vi "MPU_Stick_Read_Write_Configuration.vi"(8 "error in (no error)":errorcluster, 9 "Command":T9, 10 "Configuration Parameter":T10, 11 "MPU_Stick_Globals":T1) -> (0 "error out":errorcluster, 3 "MPU_Stick_Globals Out":T1)   [LabVIEW 2017]
uses:
  Controls/MPU_Stick_Globals.ctl
  Controls/IMU_Configuration_References.ctl
  Controls/MP_Comp_Filter_Constants_References.ctl
  Controls/MD_Threshold_References.ctl
  Controls/MD_Type_References.ctl
  Controls/LED_Configuration_References.ctl
  Controls/Primary_References.ctl
  Controls/MPU_Stick_Queues.ctl
  Controls/MPU_Stick_Queue_Element.ctl
  Controls/MPU_Stick_Queue_Commands.ctl
  Classes/ADCP.lvclass
  Controls/MPU_Stick_Config_Parameters.ctl
  Controls/MPU_Stick_Read_Write_Configurations_Command.ctl
panel:
  out "Parameter Value":string
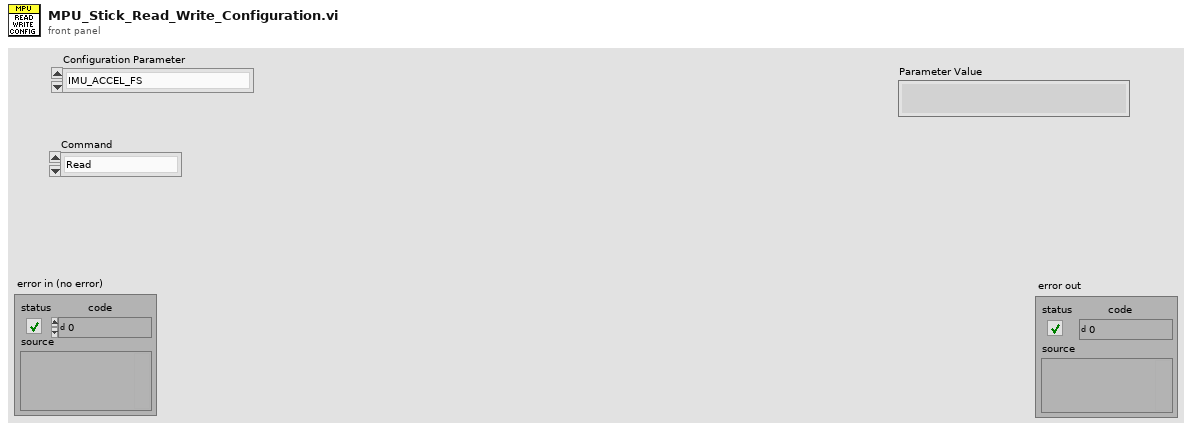
[diagram p1: front panel]
types:
  T1 = typedef "MPU_Stick_Globals.ctl" = cluster{"IMU_configuration_references":T2, "MP_Comp_Filter_Constants_References":T3, "MD_Threshold_References":T4, "MD_Type_References":T5, "LED_Configuration_References":T6, "Primary_references":T7, "MPU_Stick_Queues":T8, "ADCP":refnum<vi>}
  T2 = typedef "IMU_Configuration_References.ctl" = cluster{"Get all IMU configurations":refnum<vi>, "Set all IMU configurations":refnum<vi>, "Get sampling frequency":refnum<vi>, "Set sampling frequency":refnum<vi>, "Get calibration point count":refnum<vi>, "Set calibration point count":refnum<vi>, "Get calibration interval":refnum<vi>, "Set calibration interval":refnum<vi>, "Get Gyroscope bandwidth":refnum<vi>, "Set Gyroscope bandwidth":refnum<vi>, "Get Gyroscope F.S. Value":refnum<vi>, "Set Gyroscope F.S. Value":refnum<vi>, "Get Accelerometer bandwidth":refnum<vi>, "Set Accelerometer bandwidth":refnum<vi>, "Get Accelerometer F.S. Value":refnum<vi>, "Set Accelerometer F.S. Value":refnum<vi>, "Sampling frequency (Hz)":refnum<vi>, "Calibration point count":refnum<vi>, "Calibration interval (ms)":refnum<vi>, "IMU Gyroscope bandwidth":refnum<vi>, "IMU Gyroscope F.S. value":refnum<vi>, "IMU Accelerometer bandwidth":refnum<vi>, "IMU Accelerometer F.S. value":refnum<vi>}
  T3 = typedef "MP_Comp_Filter_Constants_References.ctl" = cluster{"Set pitch filter constant":refnum<vi>, "Get pitch filter constant":refnum<vi>, "Set roll filter constant":refnum<vi>, "Get roll filter constant":refnum<vi>, "Pitch filter constant":refnum<vi>, "Roll filter constant":refnum<vi>}
  T4 = typedef "MD_Threshold_References.ctl" = cluster{"Yaw threshold (U)":refnum<vi>, "Yaw threshold (L)":refnum<vi>, "Pitch threshold (U)":refnum<vi>, "Pitch. threshold (L)":refnum<vi>, "Roll threshold (U)":refnum<vi>, "Roll threshold (L)":refnum<vi>, "Z gyro. threshold (U)":refnum<vi>, "Z gyro. threshold (L)":refnum<vi>, "Y gyro. threshold (U)":refnum<vi>, "Y gyro. threshold (L)":refnum<vi>, "X gyro. threshold (U)":refnum<vi>, "X gyro. threshold (L)":refnum<vi>, "Z accel. threshold (U)":refnum<vi>, "Z accel. threshold (L)":refnum<vi>, "Y accel. threshold (U)":refnum<vi>, "Y accel. threshold (L)":refnum<vi>, "X accel. threshold (U)":refnum<vi>, "X accel. threshold (L)":refnum<vi>, "Set all Motion detection threshold configurations":refnum<vi>, "Get yaw threshold (upper)":refnum<vi>, "Get yaw threshold (lower)":refnum<vi>, "Get pitch threshold (upper)":refnum<vi>, "Get pitch threshold (lower)":refnum<vi>, "Get roll threshold (upper)":refnum<vi>, "Get roll threshold (lower)":refnum<vi>, "Get Z gyro threshold (upper)":refnum<vi>, "Get Z gyro threshold (lower)":refnum<vi>, "Get Y gyro threshold (upper)":refnum<vi>, "Get Y gyro threshold (lower)":refnum<vi>, "Get X gyro threshold (upper)":refnum<vi>, "Get X gyro threshold (lower)":refnum<vi>, "Get Z accel threshold (upper)":refnum<vi>, "Get Z accel threshold (lower)":refnum<vi>, "Get Y accel threshold (upper)":refnum<vi>, "Get Y accel threshold (lower)":refnum<vi>, "Get X accel threshold (upper)":refnum<vi>, "Get X accel threshold (lower)":refnum<vi>, "Get all Motion detection threshold configurations":refnum<vi>, "Set yaw threshold (upper)":refnum<vi>, "Set yaw threshold (lower)":refnum<vi>, "Set pitch threshold (upper)":refnum<vi>, "Set pitch threshold (lower)":refnum<vi>, "Set roll threshold (upper)":refnum<vi>, "Set roll threshold (lower)":refnum<vi>, "Set Z gyro threshold (upper)":refnum<vi>, "Set Z gyro threshold (lower)":refnum<vi>, "Set Y gyro threshold (upper)":refnum<vi>, "Set Y gyro threshold (lower)":refnum<vi>, "Set X gyro threshold (upper)":refnum<vi>, "Set X gyro threshold (lower)":refnum<vi>, "Set Z accel threshold (upper)":refnum<vi>, "Set Z accel threshold (lower)":refnum<vi>, "Set Y accel threshold (upper)":refnum<vi>, "Set Y accel threshold (lower)":refnum<vi>, "Set X accel threshold (upper)":refnum<vi>, "Set X accel threshold (lower)":refnum<vi>}
  T5 = typedef "MD_Type_References.ctl" = cluster{"Yaw threshold type":refnum<vi>, "Pitch threshold type":refnum<vi>, "Roll threshold type":refnum<vi>, "Z gyro threshold type":refnum<vi>, "Y gyro threshold type":refnum<vi>, "X gyro threshold type":refnum<vi>, "Z accel threshold type":refnum<vi>, "Y accel threshold type":refnum<vi>, "X accel threshold type":refnum<vi>, "Set all Motion detection type configurations":refnum<vi>, "Get all Motion detection type configurations":refnum<vi>, "Set yaw threshold type":refnum<vi>, "Get yaw threshold type":refnum<vi>, "Set pitch threshold type":refnum<vi>, "Get pitch threshold type":refnum<vi>, "Set roll threshold type":refnum<vi>, "Get roll threshold type":refnum<vi>, "Set Z gyroscope threshold type":refnum<vi>, "Get Z gyroscope threshold type":refnum<vi>, "Set Y gyroscope threshold type":refnum<vi>, "Get Y gyroscope threshold type":refnum<vi>, "Set X gyroscope threshold type":refnum<vi>, "Get X gyroscope threshold type":refnum<vi>, "Set Z accel threshold type":refnum<vi>, "Get Z accel threshold type":refnum<vi>, "Set Y accel threshold type":refnum<vi>, "Get Y accel threshold type":refnum<vi>, "Get X accel threshold type":refnum<vi>, "Set X accel threshold type":refnum<vi>}
  T6 = typedef "LED_Configuration_References.ctl" = cluster{"Get all LED configurations":refnum<vi>, "Set all LED configurations":refnum<vi>, "Get LED3 configuration":refnum<vi>, "Set LED3 configuration":refnum<vi>, "Get LED2 configuration":refnum<vi>, "Set LED2 configuration":refnum<vi>, "Get LED1 configuration":refnum<vi>, "Set LED1 configuration":refnum<vi>, "LED3 Configuration":refnum<vi>, "LED2 Configuration":refnum<vi>, "LED1 Configuration":refnum<vi>}
  T7 = typedef "Primary_References.ctl" = cluster{"3D View Image":refnum<vi>, "Plot":refnum<vi>, "Graph / 3D view tab control":refnum<vi>, "MP Reset":refnum<vi>, "Calibrate IMU":refnum<vi>, "Plot Parameter List":refnum<vi>, "Remove Parameter from Plot":refnum<vi>, "Add Parameter to Plot":refnum<vi>, "Parameter to monitor":refnum<vi>, "Yaw motion detection output":refnum<vi>, "Pitch motion detection output":refnum<vi>, "Roll motion detection output":refnum<vi>, "Z gyro motion detection output":refnum<vi>, "Y gyro motion detection output":refnum<vi>, "X gyro motion detection output":refnum<vi>, "Z accel motion detection output":refnum<vi>, "Y accel motion detection output":refnum<vi>, "X accel motion detection output":refnum<vi>, "Yaw angle (filter) (degrees)":refnum<vi>, "Pitch angle (filter) (degrees)":refnum<vi>, "Roll angle (filter) (degrees)":refnum<vi>, "Yaw angle (gyro) (degrees)":refnum<vi>, "Pitch angle (gyro) (degrees)":refnum<vi>, "Roll angle (gyro) (degrees)":refnum<vi>, "Yaw angle (accel) (degrees)":refnum<vi>, "Pitch angle (accel) (degrees)":refnum<vi>, "Roll angle (accel) (degrees)":refnum<vi>, "Z gyroscope reading (DPS)":refnum<vi>, "Y gyroscope reading (DPS)":refnum<vi>, "X gyroscope reading (DPS)":refnum<vi>, "Z accelerometer reading (G)":refnum<vi>, "Y accelerometer reading (G)":refnum<vi>, "X accelerometer reading (G)":refnum<vi>, "Save all config.":refnum<vi>, "Write all config.":refnum<vi>, "Read all config.":refnum<vi>, "Tab Control":refnum<vi>, "Baud Rate":refnum<vi>, "COM Port":refnum<vi>, "Time (ms)":refnum<vi>, "Value (Units)":refnum<vi>, "Exit Application":refnum<vi>, "Connect Device":refnum<vi>, "Progress Bar":refnum<vi>, "Get Range & Offset":refnum<vi>, "Range":refnum<vi>, "Offset":refnum<vi>, "Set Range & Offset":refnum<vi>, "Parameter name":refnum<vi>, "Plot time (ms)":refnum<vi>, "Plot value":refnum<vi>}
  T8 = typedef "MPU_Stick_Queues.ctl" = cluster{"UI Event Handler":refnum<queue>, "3D View Updater":refnum<queue>, "Plot Updater":refnum<queue>, "Serial Port Reader":refnum<queue>, "UI Indicators Updater":refnum<queue>}
  T9 = typedef "MPU_Stick_Read_Write_Configurations_Command.ctl" = enum16{"Read", "Write", "Write All", "Read All"}
  T10 = typedef "MPU_Stick_Config_Parameters.ctl" = enum16{"IMU_ACCEL_FS", "IMU_ACCEL_BW", "IMU_GYRO_FS", "IMU_GYRO_BW", "IMU_CALIB_INTERVAL", "IMU_CALIB_POINT_COUNT", "IMU_SAMPLING_FREQ", "LED1_CONFIG", "LED2_CONFIG", "LED3_CONFIG", "MP_ROLL_FILTER_CONSTANT", "MP_PITCH_FILTER_CONSTANT", "MP_THRESHOLD_X_ACCEL_LOW", "MP_THRESHOLD_X_ACCEL_HIGH", "MP_THRESHOLD_Y_ACCEL_LOW", "MP_THRESHOLD_Y_ACCEL_HIGH", "MP_THRESHOLD_Z_ACCEL_LOW", "MP_THRESHOLD_Z_ACCEL_HIGH", "MP_THRESHOLD_X_GYRO_LOW", "MP_THRESHOLD_X_GYRO_HIGH", "MP_THRESHOLD_Y_GYRO_LOW", "MP_THRESHOLD_Y_GYRO_HIGH", "MP_THRESHOLD_Z_GYRO_LOW", "MP_THRESHOLD_Z_GYRO_HIGH", "MP_THRESHOLD_ROLL_LOW", "MP_THRESHOLD_ROLL_HIGH", "MP_THRESHOLD_PITCH_LOW", "MP_THRESHOLD_PITCH_HIGH", "MP_THRESHOLD_YAW_LOW", "MP_THRESHOLD_YAW_HIGH", "MP_DETECTION_TYPE_X_ACCEL", "MP_DETECTION_TYPE_Y_ACCEL", "MP_DETECTION_TYPE_Z_ACCEL", "MP_DETECTION_TYPE_X_GYRO", "MP_DETECTION_TYPE_Y_GYRO", "MP_DETECTION_TYPE_Z_GYRO", "MP_DETECTION_TYPE_ROLL", "MP_DETECTION_TYPE_PITCH", "MP_DETECTION_TYPE_YAW"}
  T11 = cluster{"Parameter name":string, "Node name":string, "Node ID":u8, "Frame name":string, "Frame ID":u8, "Start bit":u32, "Bit length":u32, "Factor":dbl, "Offset":dbl, "Minimum":dbl, "Maximum":dbl, "Value":string, "Comments":string, "Data_Type":enum16{"BOOL", "UNSIGNED", "SIGNED", "FLOAT32", "ENUM"}, "Enum List":string[]}[]
  T12 = typedef "IMU_Accelerometer_Full_Scale_Values.ctl" = enum16{"2G", "4G", "8G", "16G"}
  T13 = typedef "IMU_Accelerometer_Bandwidth.ctl" = enum16{"IMU_ACCEL_BW_460_Hz", "IMU_ACCEL_BW_184_Hz", "IMU_ACCEL_BW_92_Hz", "IMU_ACCEL_BW_41_Hz", "IMU_ACCEL_BW_20_Hz", "IMU_ACCEL_BW_10_Hz", "IMU_ACCEL_BW_5_Hz"}
  T14 = typedef "IMU_Gyroscope_Full_Scale_Values.ctl" = enum16{"250 DPS", "500 DPS", "1000 DPS", "2000 DPS"}
  T15 = typedef "IMU_Gyroscope_Bandwidth.ctl" = enum16{"IMU_GYRO_BW_NONE", "IMU_GYRO_BW_184_Hz", "IMU_GYRO_BW_92_Hz", "IMU_GYRO_BW_41_Hz", "IMU_GYRO_BW_20_Hz", "IMU_GYRO_BW_10_Hz", "IMU_GYRO_BW_5_Hz"}
  T16 = typedef "LED_config.ctl" = enum16{"UC_DIGITAL_OUTPUT", "X_ACCEL_PWM", "Y_ACCEL_PWM", "Z_ACCEL_PWM", "X_ACCEL_MD_OUTPUT", "Y_ACCEL_MD_OUTPUT", "Z_ACCEL_MD_OUTPUT", "X_GYRO_PWM", "Y_GYRO_PWM", "Z_GYRO_PWM", "X_GYRO_MD_OUTPUT", "Y_GYRO_MD_OUTPUT", "Z_GYRO_MD_OUTPUT", "ROLL_PWM_OUTPUT", "PITCH_PWM_OUTPUT", "YAW_PWM_OUTPUT", "ROLL_MD_OUTPUT", "PITCH_MD_OUTPUT", "YAW_MD_OUTPUT", "UC_PWM_OUTPUT"}
  T17 = typedef "Motion_Detection_Threshold_Type.ctl" = enum16{"ABS_LESSER_THAN", "ABS_GREATER_THAN", "LESSER_THAN", "GREATER_THAN", "WINDOWED_MODE_WITHIN_BOUNDS", "WINDOWED_MODE_OUTSIDE_BOUNDS"}
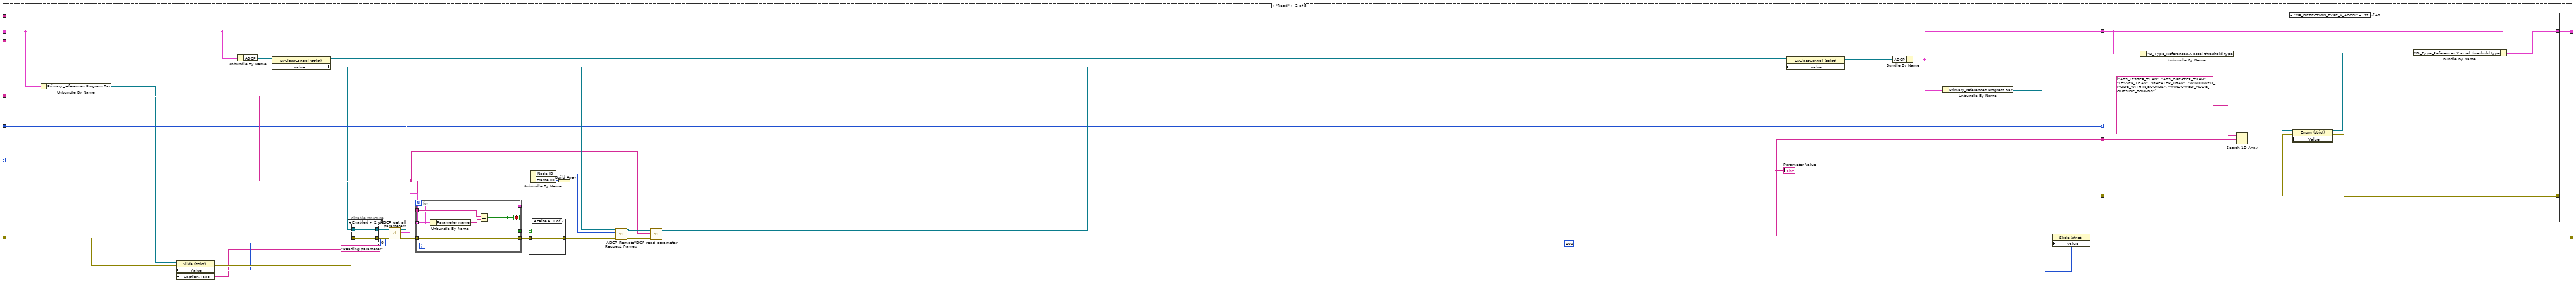
[diagram p4: hidden frame]
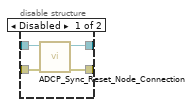
[diagram p5: hidden frame]
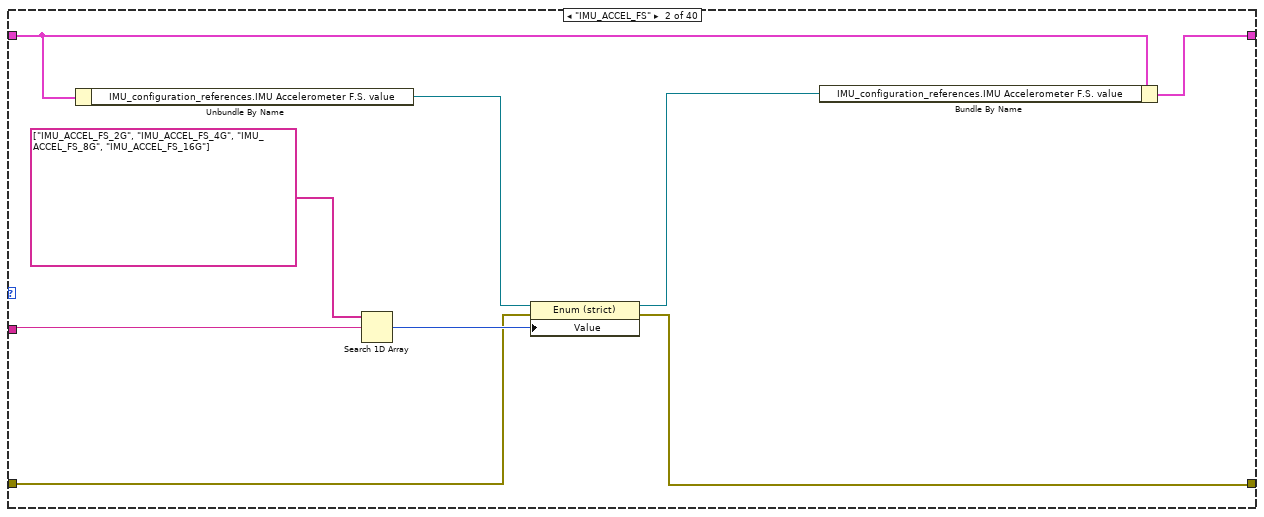
[diagram p8: hidden frame]
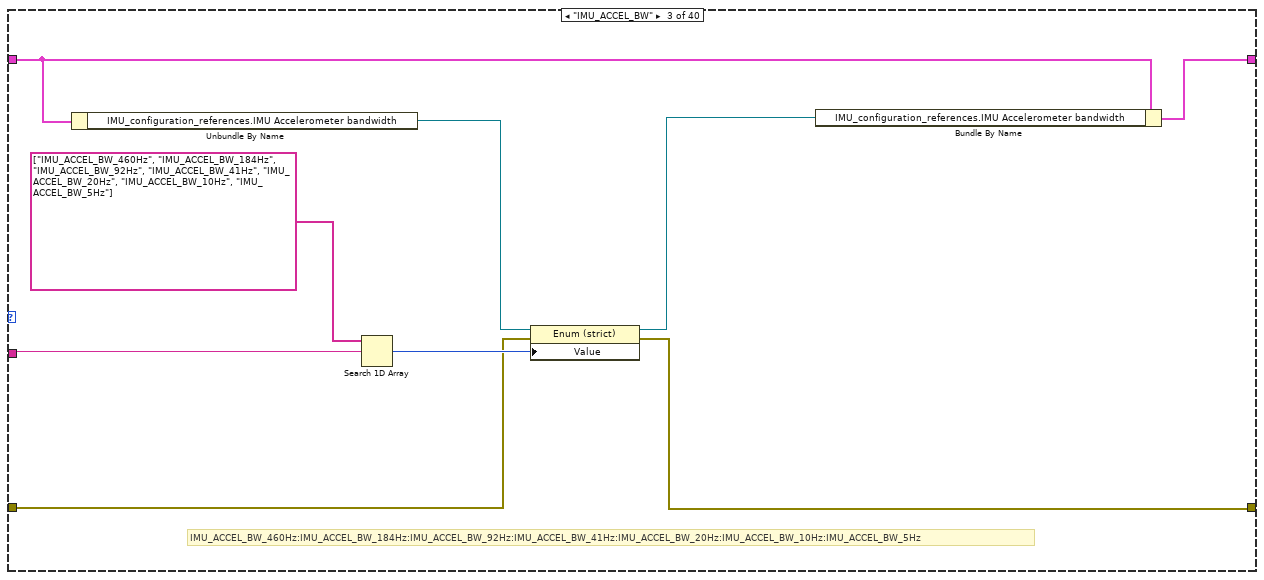
[diagram p9: hidden frame]
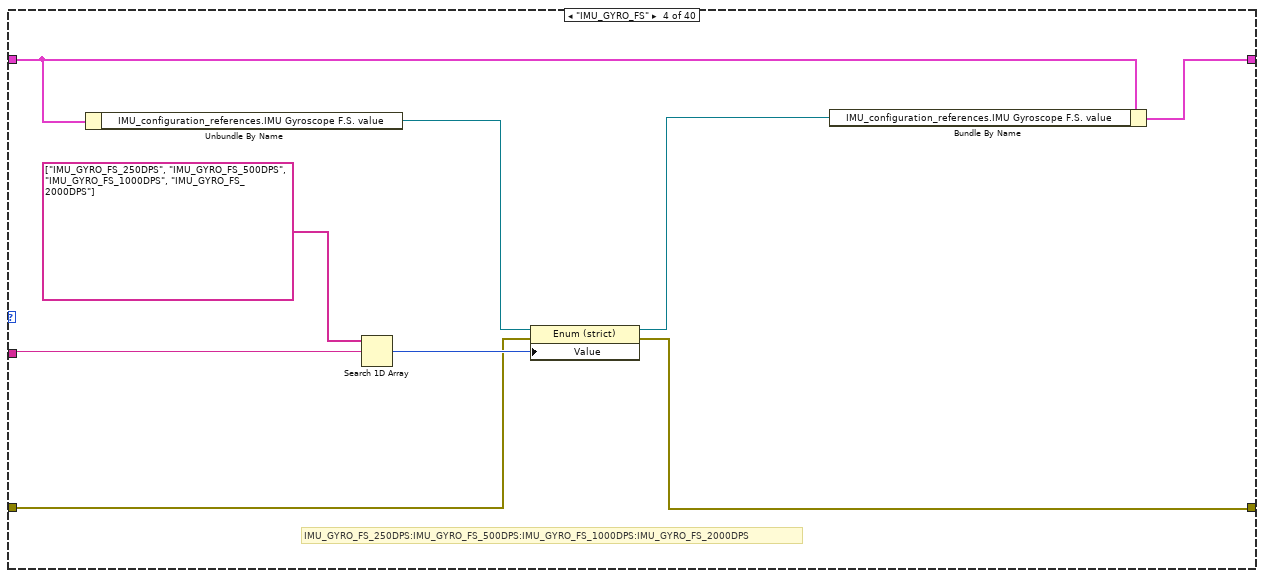
[diagram p10: hidden frame]
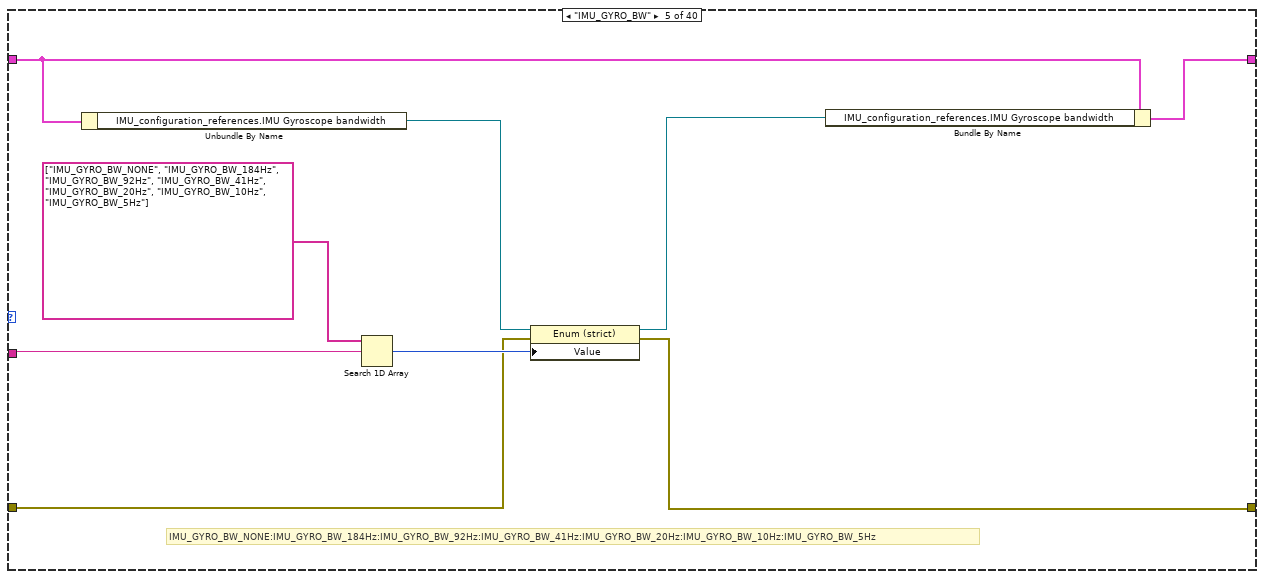
[diagram p11: hidden frame]
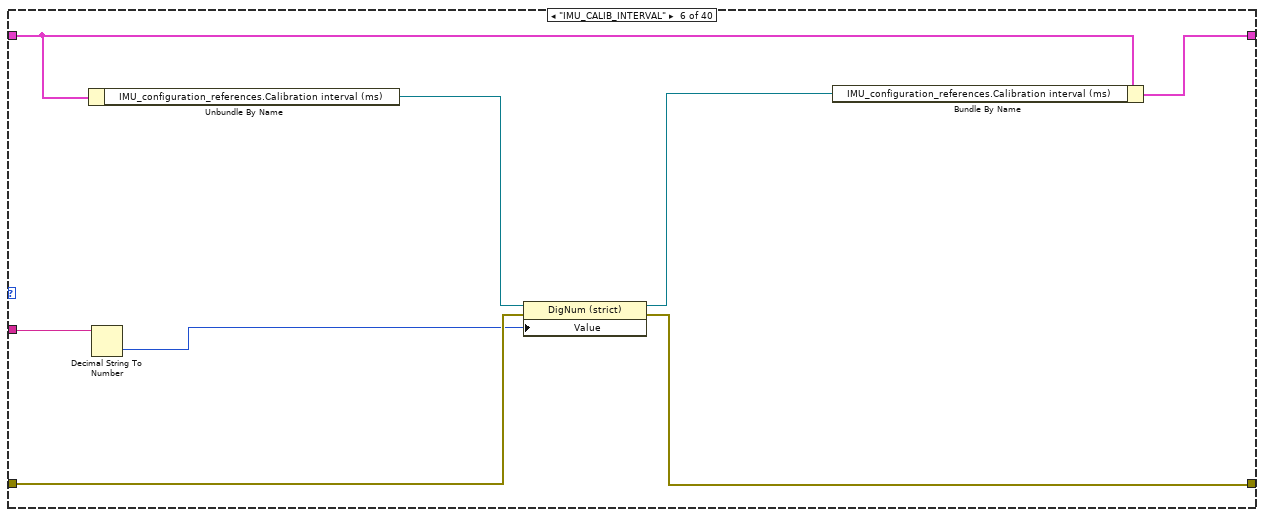
[diagram p12: hidden frame]
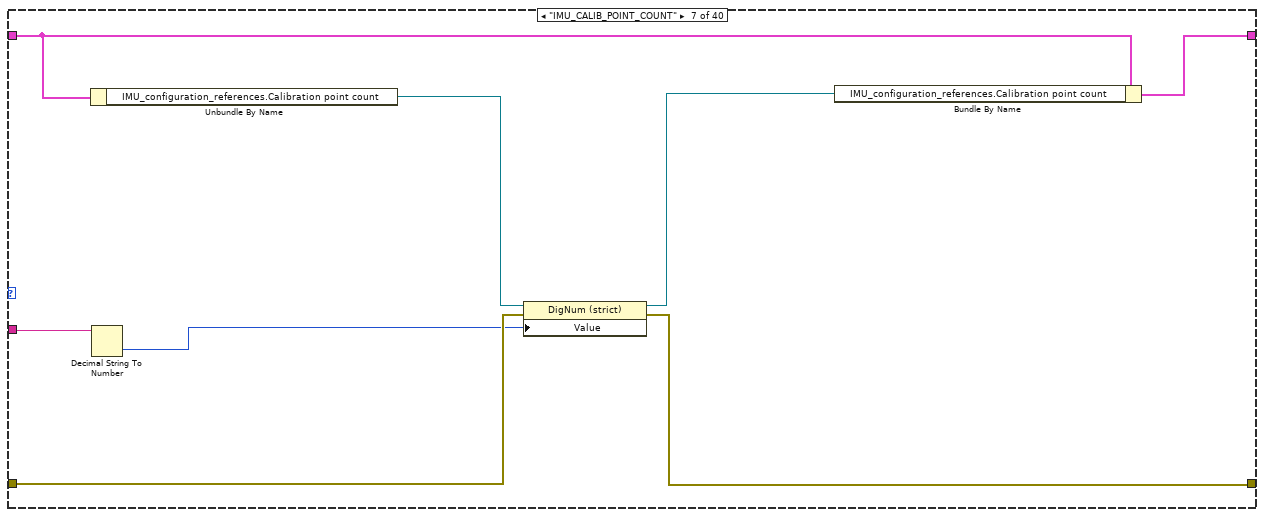
[diagram p13: hidden frame]
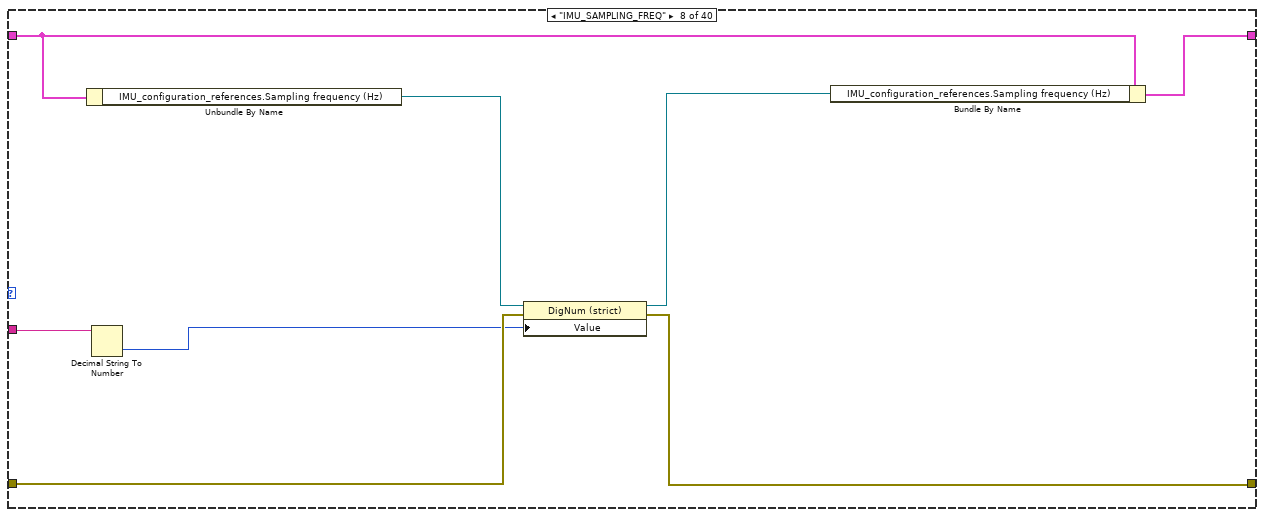
[diagram p14: hidden frame]
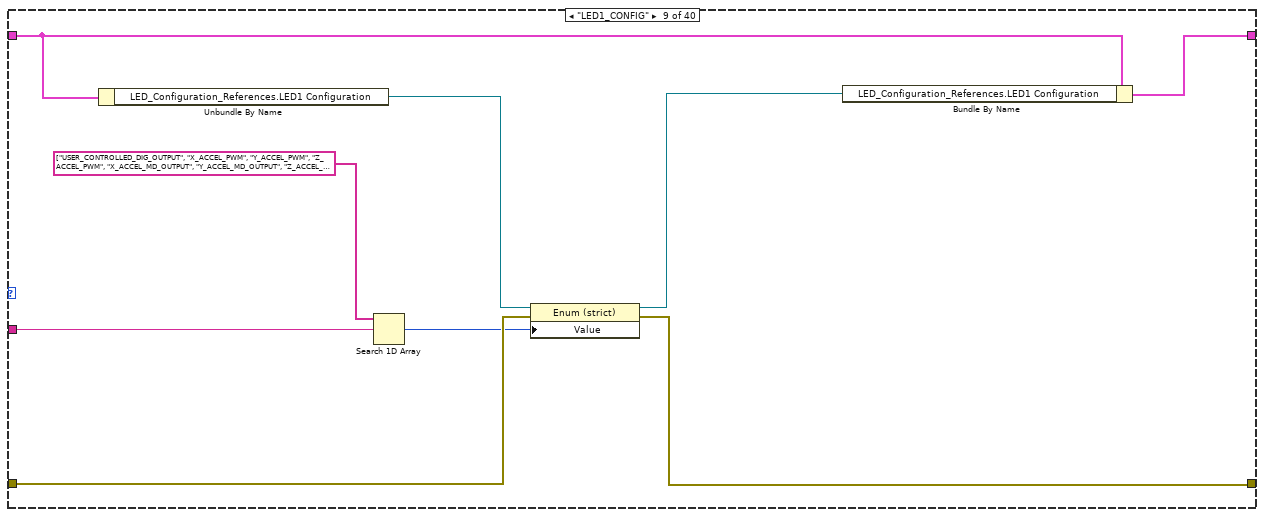
[diagram p15: hidden frame]
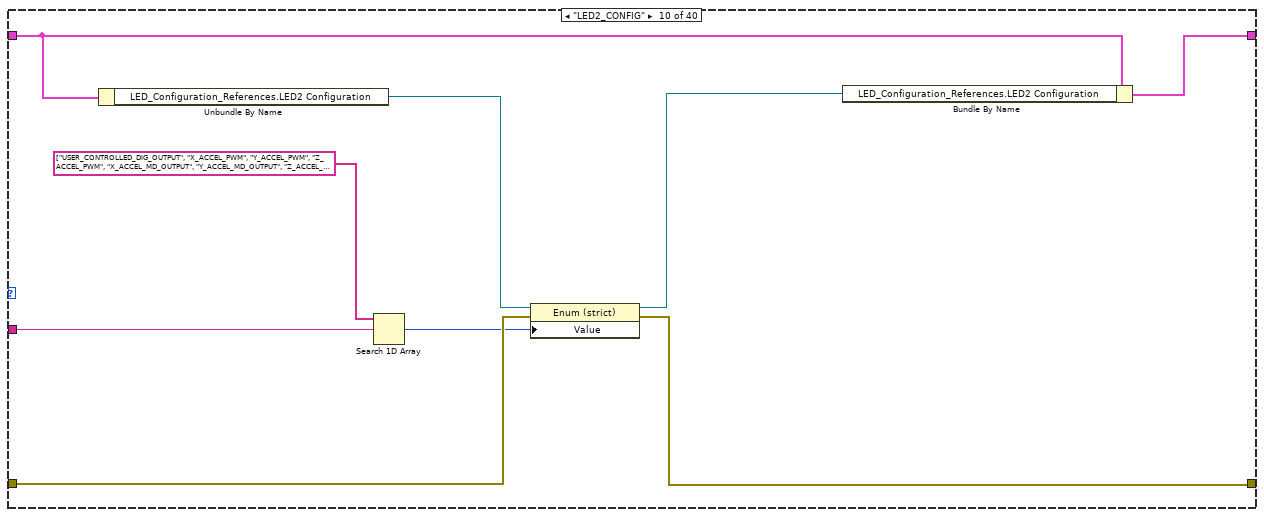
[diagram p16: hidden frame]
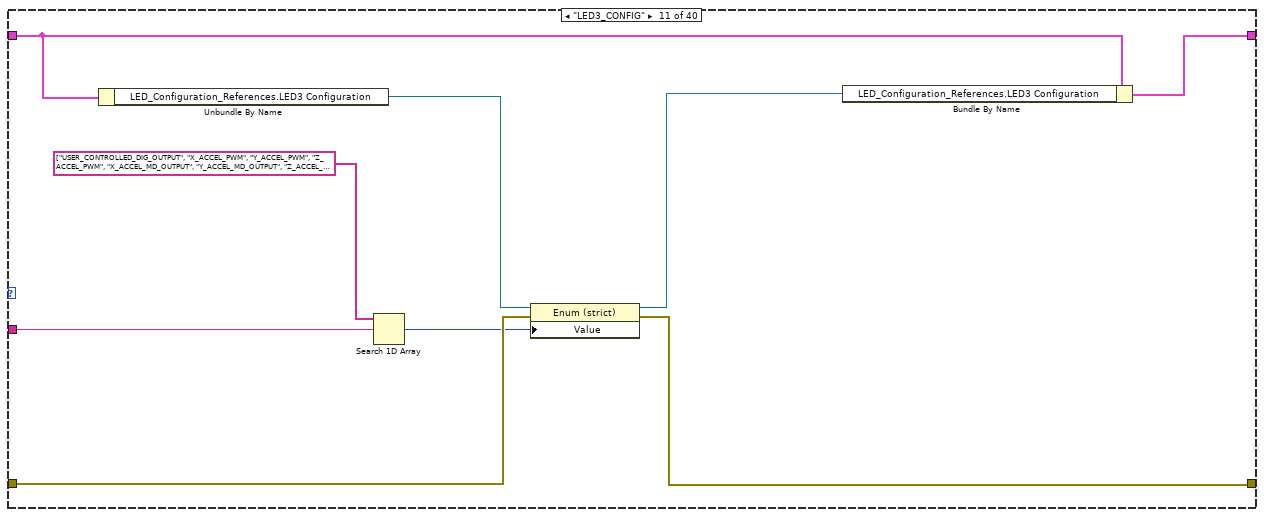
[diagram p17: hidden frame]
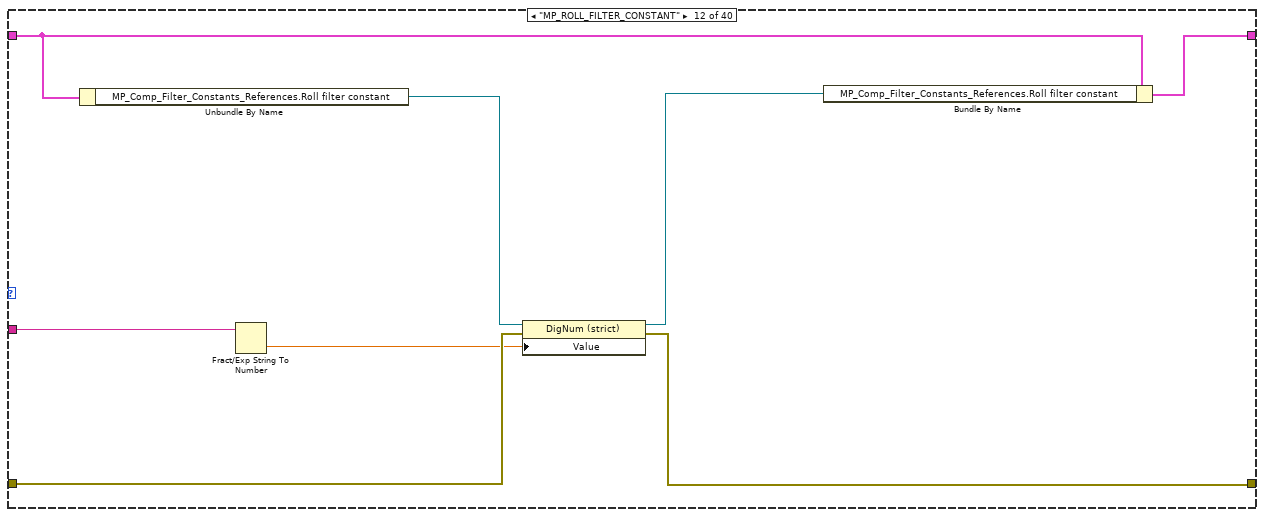
[diagram p18: hidden frame]
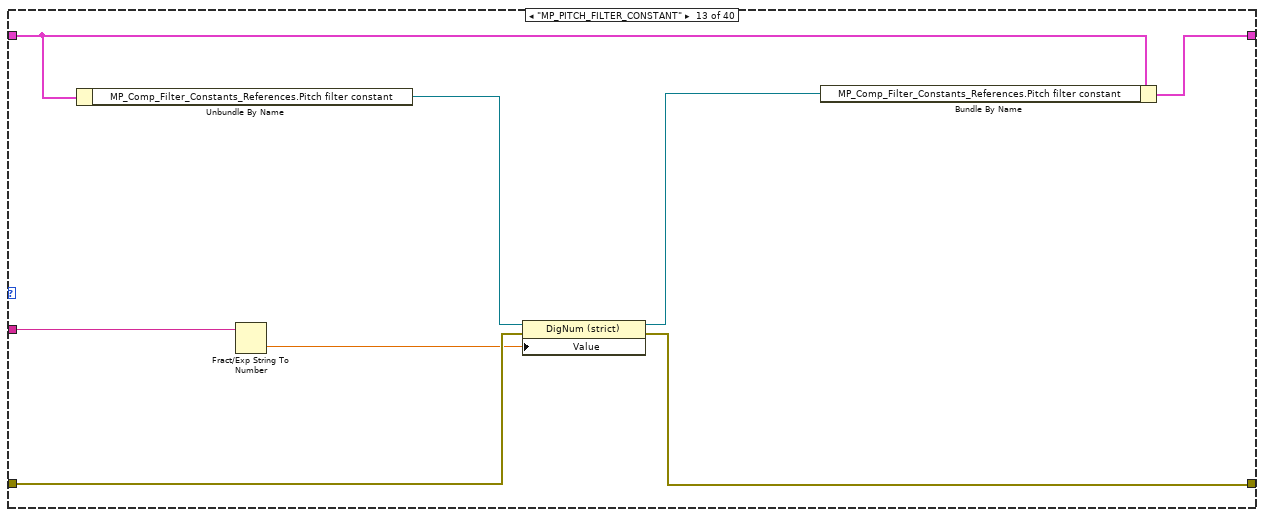
[diagram p19: hidden frame]
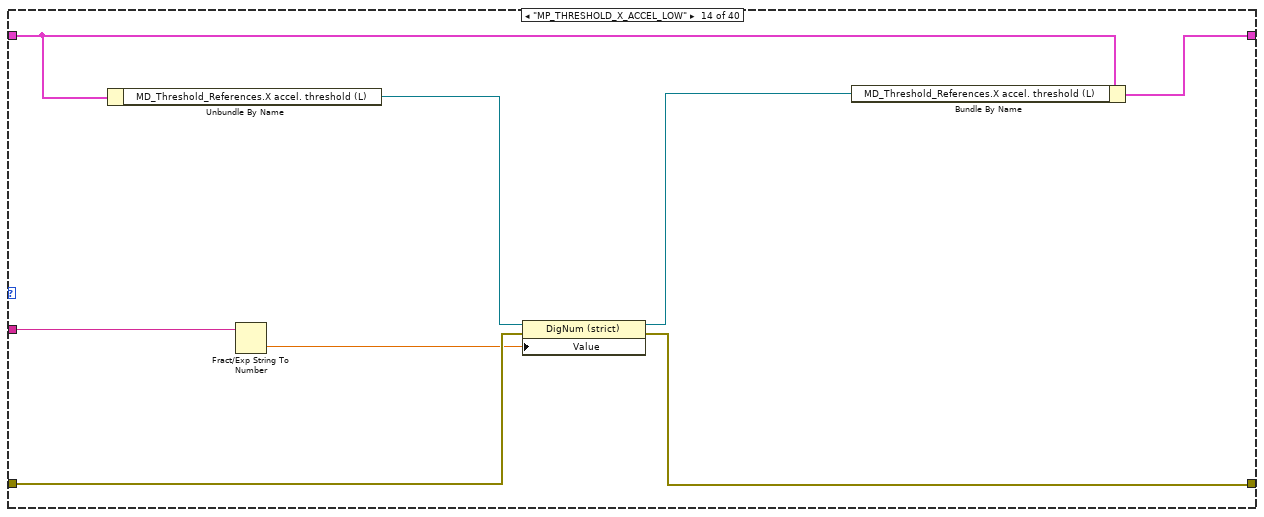
[diagram p20: hidden frame]
diagram:
  (unwired) string[] ["MPU_STICK:IMU_CONFIG_WRITE_ENABLE:IMU_CONFIG_ACCEL_FS_WE", "MPU_STICK:IMU_CONFIG_WRITE_ENABLE:IMU_CONFIG_ACCEL_BW_WE", "MPU_STICK:IMU_CONFIG_WRITE_ENABLE:IMU_CONFIG_GYRO_FS_WE", "MPU_STICK:IMU_CONFIG_WRITE_ENABLE:IMU_CONFIG_GYRO_BW_WE", "MPU_STICK:IMU_CONFIG_WRITE_ENABLE:IMU_CONFIG_CALIB_INTERVAL_WE", "MPU_STICK:IMU_CONFIG_WRITE_ENABLE:IMU_CONFIG_CALIB_POINTS_WE", "MPU_STICK:IMU_CONFIG_WRITE_ENABLE:IMU_CONFIG_SAMPLING_RATE_WE", "MPU_STICK:LED_MODE_CONFIG:LED1_MODE_WE", "MPU_STICK:LED_MODE_CONFIG:LED2_MODE_WE", "MPU_STICK:LED_MODE_CONFIG:LED3_MODE_WE", "MPU_STICK:MD_WRITE_CONFIG:MP_ROLL_FILTER_CONSTANT_WE", "MPU_STICK:MD_WRITE_CONFIG:MP_PITCH_FILTER_CONSTANT_WE", "MPU_STICK:MD_WRITE_CONFIG:MD_ACCEL_X_THRESHOLD_LOW_WE", "MPU_STICK:MD_WRITE_CONFIG:MD_ACCEL_X_THRESHOLD_HIGH_WE", "MPU_STICK:MD_WRITE_CONFIG:MD_ACCEL_Y_THRESHOLD_LOW_WE", "MPU_STICK:MD_WRITE_CONFIG:MD_ACCEL_Y_THRESHOLD_HIGH_WE", "MPU_STICK:MD_WRITE_CONFIG:MD_ACCEL_Z_THRESHOLD_LOW_WE", "MPU_STICK:MD_WRITE_CONFIG:MD_ACCEL_Z_THRESHOLD_HIGH_WE", "MPU_STICK:MD_WRITE_CONFIG:MD_GYRO_X_THRESHOLD_LOW_WE", "MPU_STICK:MD_WRITE_CONFIG:MD_GYRO_X_THRESHOLD_HIGH_WE", "MPU_STICK:MD_WRITE_CONFIG:MD_GYRO_Y_THRESHOLD_LOW_WE", "MPU_STICK:MD_WRITE_CONFIG:MD_GYRO_Y_THRESHOLD_HIGH_WE", "MPU_STICK:MD_WRITE_CONFIG:MD_GYRO_Z_THRESHOLD_LOW_WE", "MPU_STICK:MD_WRITE_CONFIG:MD_GYRO_Z_THRESHOLD_HIGH_WE", "MPU_STICK:MD_WRITE_CONFIG:MD_ROLL_THRESHOLD_LOW_WE", "MPU_STICK:MD_WRITE_CONFIG:MD_ROLL_THRESHOLD_HIGH_WE", "MPU_STICK:MD_WRITE_CONFIG:MD_PITCH_THRESHOLD_LOW_WE", "MPU_STICK:MD_WRITE_CONFIG:MD_PITCH_THRESHOLD_HIGH_WE", "MPU_STICK:MD_WRITE_CONFIG:MD_YAW_THRESHOLD_LOW_WE", "MPU_STICK:MD_WRITE_CONFIG:MD_YAW_THRESHOLD_HIGH_WE", "MPU_STICK:MD_WRITE_CONFIG:MD_ACCEL_X_THRESHOLD_TYPE_WE", "MPU_STICK:MD_WRITE_CONFIG:MD_ACCEL_Y_THRESHOLD_TYPE_WE", "MPU_STICK:MD_WRITE_CONFIG:MD_ACCEL_Z_THRESHOLD_TYPE_WE", "MPU_STICK:MD_WRITE_CONFIG:MD_GYRO_X_THRESHOLD_TYPE_WE", "MPU_STICK:MD_WRITE_CONFIG:MD_GYRO_Y_THRESHOLD_TYPE_WE", "MPU_STICK:MD_WRITE_CONFIG:MD_GYRO_Z_THRESHOLD_TYPE_WE", "MPU_STICK:MD_WRITE_CONFIG:MD_ROLL_THRESHOLD_TYPE_WE", "MPU_STICK:MD_WRITE_CONFIG:MD_PITCH_THRESHOLD_TYPE_WE", "MPU_STICK:MD_WRITE_CONFIG:MD_YAW_THRESHOLD_TYPE_WE"]  # MPU Stick Configuration Write Enable Bit Names
  (unwired) string[] ["MPU_STICK:IMU_CONFIG_REG_B:IMU_CONFIG_ACCEL_FS", "MPU_STICK:IMU_CONFIG_REG_B:IMU_CONFIG_ACCEL_BW", "MPU_STICK:IMU_CONFIG_REG_B:IMU_CONFIG_GYRO_FS", "MPU_STICK:IMU_CONFIG_REG_B:IMU_CONFIG_GYRO_BW", "MPU_STICK:IMU_CONFIG_REG_A:IMU_CONFIG_CALIB_INTERVAL", "MPU_STICK:IMU_CONFIG_REG_A:IMU_CONFIG_CALIB_POINTS", "MPU_STICK:IMU_CONFIG_REG_A:IMU_CONFIG_SAMPLING_RATE", "MPU_STICK:LED_MODE_CONFIG:LED1_MODE", "MPU_STICK:LED_MODE_CONFIG:LED2_MODE", "MPU_STICK:LED_MODE_CONFIG:LED3_MODE", "MPU_STICK:MP_ROLL_FILTER_CONSTANT:MP_ROLL_FILTER_CONSTANT", "MPU_STICK:MP_PITCH_FILTER_CONSTANT:MP_PITCH_FILTER_CONSTANT", "MPU_STICK:MD_ACCEL_X_THRESHOLD_LOW:MD_ACCEL_X_THRESHOLD_LOW", "MPU_STICK:MD_ACCEL_X_THRESHOLD_HIGH:MD_ACCEL_X_THRESHOLD_HIGH", "MPU_STICK:MD_ACCEL_Y_THRESHOLD_LOW:MD_ACCEL_Y_THRESHOLD_LOW", "MPU_STICK:MD_ACCEL_Y_THRESHOLD_HIGH:MD_ACCEL_Y_THRESHOLD_HIGH", "MPU_STICK:MD_ACCEL_Z_THRESHOLD_LOW:MD_ACCEL_Z_THRESHOLD_LOW", "MPU_STICK:MD_ACCEL_Z_THRESHOLD_HIGH:MD_ACCEL_Z_THRESHOLD_HIGH", "MPU_STICK:MD_GYRO_X_THRESHOLD_LOW:MD_GYRO_X_THRESHOLD_LOW", "MPU_STICK:MD_GYRO_X_THRESHOLD_HIGH:MD_GYRO_X_THRESHOLD_HIGH", "MPU_STICK:MD_GYRO_Y_THRESHOLD_LOW:MD_GYRO_Y_THRESHOLD_LOW", "MPU_STICK:MD_GYRO_Y_THRESHOLD_HIGH:MD_GYRO_Y_THRESHOLD_HIGH", "MPU_STICK:MD_GYRO_Z_THRESHOLD_LOW:MD_GYRO_Z_THRESHOLD_LOW", "MPU_STICK:MD_GYRO_Z_THRESHOLD_HIGH:MD_GYRO_Z_THRESHOLD_HIGH", "MPU_STICK:MD_ROLL_THRESHOLD_LOW:MD_ROLL_THRESHOLD_LOW", "MPU_STICK:MD_ROLL_THRESHOLD_HIGH:MD_ROLL_THRESHOLD_HIGH", "MPU_STICK:MD_PITCH_THRESHOLD_LOW:MD_PITCH_THRESHOLD_LOW", "MPU_STICK:MD_PITCH_THRESHOLD_HIGH:MD_PITCH_THRESHOLD_HIGH", "MPU_STICK:MD_YAW_THRESHOLD_LOW:MD_YAW_THRESHOLD_LOW", "MPU_STICK:MD_YAW_THRESHOLD_HIGH:MD_YAW_THRESHOLD_HIGH", "MPU_STICK:MD_THRESHOLD_TYPE:MD_ACCEL_X_THRESHOLD_TYPE", "MPU_STICK:MD_THRESHOLD_TYPE:MD_ACCEL_Y_THRESHOLD_TYPE", "MPU_STICK:MD_THRESHOLD_TYPE:MD_ACCEL_Z_THRESHOLD_TYPE", "MPU_STICK:MD_THRESHOLD_TYPE:MD_GYRO_X_THRESHOLD_TYPE", "MPU_STICK:MD_THRESHOLD_TYPE:MD_GYRO_Y_THRESHOLD_TYPE", "MPU_STICK:MD_THRESHOLD_TYPE:MD_GYRO_Z_THRESHOLD_TYPE", "MPU_STICK:MD_THRESHOLD_TYPE:MD_ROLL_THRESHOLD_TYPE", "MPU_STICK:MD_THRESHOLD_TYPE:MD_PITCH_THRESHOLD_TYPE", "MPU_STICK:MD_THRESHOLD_TYPE:MD_YAW_THRESHOLD_TYPE"]  # MPU Stick Configuration Parameters
  (unwired) string[] ["MPU_STICK:IMU_CONFIG_WRITE_ENABLE:IMU_CONFIG_SAMPLING_RATE_WE", "MPU_STICK:IMU_CONFIG_WRITE_ENABLE:IMU_CONFIG_CALIB_INTERVAL_WE", "MPU_STICK:IMU_CONFIG_WRITE_ENABLE:IMU_CONFIG_CALIB_POINTS_WE", "MPU_STICK:IMU_CONFIG_WRITE_ENABLE:IMU_CONFIG_GYRO_BW_WE", "MPU_STICK:IMU_CONFIG_WRITE_ENABLE:IMU_CONFIG_ACCEL_BW_WE", "MPU_STICK:IMU_CONFIG_WRITE_ENABLE:IMU_CONFIG_GYRO_FS_WE", "MPU_STICK:IMU_CONFIG_WRITE_ENABLE:IMU_CONFIG_ACCEL_FS_WE", "MPU_STICK:MD_WRITE_CONFIG:MD_ACCEL_X_THRESHOLD_LOW_WE", "MPU_STICK:MD_WRITE_CONFIG:MD_ACCEL_X_THRESHOLD_HIGH_WE", "MPU_STICK:MD_WRITE_CONFIG:MD_ACCEL_Y_THRESHOLD_LOW_WE", "MPU_STICK:MD_WRITE_CONFIG:MD_ACCEL_Y_THRESHOLD_HIGH_WE", "MPU_STICK:MD_WRITE_CONFIG:MD_ACCEL_Z_THRESHOLD_LOW_WE", "MPU_STICK:MD_WRITE_CONFIG:MD_ACCEL_Z_THRESHOLD_HIGH_WE", "MPU_STICK:MD_WRITE_CONFIG:MD_GYRO_X_THRESHOLD_LOW_WE", "MPU_STICK:MD_WRITE_CONFIG:MD_GYRO_X_THRESHOLD_HIGH_WE", "MPU_STICK:MD_WRITE_CONFIG:MD_GYRO_Y_THRESHOLD_LOW_WE", "MPU_STICK:MD_WRITE_CONFIG:MD_GYRO_Y_THRESHOLD_HIGH_WE", "MPU_STICK:MD_WRITE_CONFIG:MD_GYRO_Z_THRESHOLD_LOW_WE", "MPU_STICK:MD_WRITE_CONFIG:MD_GYRO_Z_THRESHOLD_HIGH_WE", "MPU_STICK:MD_WRITE_CONFIG:MD_ROLL_THRESHOLD_LOW_WE", "MPU_STICK:MD_WRITE_CONFIG:MD_ROLL_THRESHOLD_HIGH_WE", "MPU_STICK:MD_WRITE_CONFIG:MD_PITCH_THRESHOLD_LOW_WE", "MPU_STICK:MD_WRITE_CONFIG:MD_PITCH_THRESHOLD_HIGH_WE", "MPU_STICK:MD_WRITE_CONFIG:MD_YAW_THRESHOLD_LOW_WE", "MPU_STICK:MD_WRITE_CONFIG:MD_YAW_THRESHOLD_HIGH_WE", "MPU_STICK:MD_WRITE_CONFIG:MP_ROLL_FILTER_CONSTANT_WE", "MPU_STICK:MD_WRITE_CONFIG:MP_PITCH_FILTER_CONSTANT_WE", "MPU_STICK:MD_WRITE_CONFIG:MP_YAW_FILTER_CONSTANT_WE", "MPU_STICK:MD_WRITE_CONFIG:MD_ACCEL_X_THRESHOLD_TYPE_WE", "MPU_STICK:MD_WRITE_CONFIG:MD_ACCEL_Y_THRESHOLD_TYPE_WE", "MPU_STICK:MD_WRITE_CONFIG:MD_ACCEL_Z_THRESHOLD_TYPE_WE", "MPU_STICK:MD_WRITE_CONFIG:MD_GYRO_X_THRESHOLD_TYPE_WE", "MPU_STICK:MD_WRITE_CONFIG:MD_GYRO_Y_THRESHOLD_TYPE_WE", "MPU_STICK:MD_WRITE_CONFIG:MD_GYRO_Z_THRESHOLD_TYPE_WE", "MPU_STICK:MD_WRITE_CONFIG:MD_ROLL_THRESHOLD_TYPE_WE", "MPU_STICK:MD_WRITE_CONFIG:MD_PITCH_THRESHOLD_TYPE_WE", "MPU_STICK:MD_WRITE_CONFIG:MD_YAW_THRESHOLD_TYPE_WE", "MPU_STICK:LED_MODE_CONFIG:LED1_MODE_WE", "MPU_STICK:LED_MODE_CONFIG:LED2_MODE_WE", "MPU_STICK:LED_MODE_CONFIG:LED3_MODE_WE", "MPU_STICK:LED_UC_WRITE:LED_UC_STATE_WE", "MPU_STICK:LED_UC_WRITE:LED_UC_DUTY_WE"] ("Array")
  n1 = while {
    shift-right: [w14] -> w1
    shift-left: "MPU_Stick_Globals" -> [w15]
    tunnel: "Configuration Parameter" -> [w8]
    tunnel: "error in (no error)" -> [w13]
    tunnel: "Command" -> [w16]
    tunnel: [w12] -> w2
    stop <- TRUE stop-if-true
    w9 = string[] ["MPU_STICK:IMU_CONFIG_WRITE_ENABLE:IMU_CONFIG_ACCEL_FS_WE", "MPU_STICK:IMU_CONFIG_WRITE_ENABLE:IMU_CONFIG_ACCEL_BW_WE", "MPU_STICK:IMU_CONFIG_WRITE_ENABLE:IMU_CONFIG_GYRO_FS_WE", "MPU_STICK:IMU_CONFIG_WRITE_ENABLE:IMU_CONFIG_GYRO_BW_WE", "MPU_STICK:IMU_CONFIG_WRITE_ENABLE:IMU_CONFIG_CALIB_INTERVAL_WE", "MPU_STICK:IMU_CONFIG_WRITE_ENABLE:IMU_CONFIG_CALIB_POINTS_WE", "MPU_STICK:IMU_CONFIG_WRITE_ENABLE:IMU_CONFIG_SAMPLING_RATE_WE", "MPU_STICK:LED_MODE_CONFIG:LED1_MODE_WE", "MPU_STICK:LED_MODE_CONFIG:LED2_MODE_WE", "MPU_STICK:LED_MODE_CONFIG:LED3_MODE_WE", "MPU_STICK:MD_WRITE_CONFIG:MP_ROLL_FILTER_CONSTANT_WE", "MPU_STICK:MD_WRITE_CONFIG:MP_PITCH_FILTER_CONSTANT_WE", "MPU_STICK:MD_WRITE_CONFIG:MD_ACCEL_X_THRESHOLD_LOW_WE", "MPU_STICK:MD_WRITE_CONFIG:MD_ACCEL_X_THRESHOLD_HIGH_WE", "MPU_STICK:MD_WRITE_CONFIG:MD_ACCEL_Y_THRESHOLD_LOW_WE", "MPU_STICK:MD_WRITE_CONFIG:MD_ACCEL_Y_THRESHOLD_HIGH_WE", "MPU_STICK:MD_WRITE_CONFIG:MD_ACCEL_Z_THRESHOLD_LOW_WE", "MPU_STICK:MD_WRITE_CONFIG:MD_ACCEL_Z_THRESHOLD_HIGH_WE", "MPU_STICK:MD_WRITE_CONFIG:MD_GYRO_X_THRESHOLD_LOW_WE", "MPU_STICK:MD_WRITE_CONFIG:MD_GYRO_X_THRESHOLD_HIGH_WE", "MPU_STICK:MD_WRITE_CONFIG:MD_GYRO_Y_THRESHOLD_LOW_WE", "MPU_STICK:MD_WRITE_CONFIG:MD_GYRO_Y_THRESHOLD_HIGH_WE", "MPU_STICK:MD_WRITE_CONFIG:MD_GYRO_Z_THRESHOLD_LOW_WE", "MPU_STICK:MD_WRITE_CONFIG:MD_GYRO_Z_THRESHOLD_HIGH_WE", "MPU_STICK:MD_WRITE_CONFIG:MD_ROLL_THRESHOLD_LOW_WE", "MPU_STICK:MD_WRITE_CONFIG:MD_ROLL_THRESHOLD_HIGH_WE", "MPU_STICK:MD_WRITE_CONFIG:MD_PITCH_THRESHOLD_LOW_WE", "MPU_STICK:MD_WRITE_CONFIG:MD_PITCH_THRESHOLD_HIGH_WE", "MPU_STICK:MD_WRITE_CONFIG:MD_YAW_THRESHOLD_LOW_WE", "MPU_STICK:MD_WRITE_CONFIG:MD_YAW_THRESHOLD_HIGH_WE", "MPU_STICK:MD_WRITE_CONFIG:MD_ACCEL_X_THRESHOLD_TYPE_WE", "MPU_STICK:MD_WRITE_CONFIG:MD_ACCEL_Y_THRESHOLD_TYPE_WE", "MPU_STICK:MD_WRITE_CONFIG:MD_ACCEL_Z_THRESHOLD_TYPE_WE", "MPU_STICK:MD_WRITE_CONFIG:MD_GYRO_X_THRESHOLD_TYPE_WE", "MPU_STICK:MD_WRITE_CONFIG:MD_GYRO_Y_THRESHOLD_TYPE_WE", "MPU_STICK:MD_WRITE_CONFIG:MD_GYRO_Z_THRESHOLD_TYPE_WE", "MPU_STICK:MD_WRITE_CONFIG:MD_ROLL_THRESHOLD_TYPE_WE", "MPU_STICK:MD_WRITE_CONFIG:MD_PITCH_THRESHOLD_TYPE_WE", "MPU_STICK:MD_WRITE_CONFIG:MD_YAW_THRESHOLD_TYPE_WE"]  # MPU Stick Configuration Write Enable Bit Names
    w10 = string[] ["MPU_STICK:IMU_CONFIG_REG_B:IMU_CONFIG_ACCEL_FS", "MPU_STICK:IMU_CONFIG_REG_B:IMU_CONFIG_ACCEL_BW", "MPU_STICK:IMU_CONFIG_REG_B:IMU_CONFIG_GYRO_FS", "MPU_STICK:IMU_CONFIG_REG_B:IMU_CONFIG_GYRO_BW", "MPU_STICK:IMU_CONFIG_REG_A:IMU_CONFIG_CALIB_INTERVAL", "MPU_STICK:IMU_CONFIG_REG_A:IMU_CONFIG_CALIB_POINTS", "MPU_STICK:IMU_CONFIG_REG_A:IMU_CONFIG_SAMPLING_RATE", "MPU_STICK:LED_MODE_CONFIG:LED1_MODE", "MPU_STICK:LED_MODE_CONFIG:LED2_MODE", "MPU_STICK:LED_MODE_CONFIG:LED3_MODE", "MPU_STICK:MP_ROLL_FILTER_CONSTANT:MP_ROLL_FILTER_CONSTANT", "MPU_STICK:MP_PITCH_FILTER_CONSTANT:MP_PITCH_FILTER_CONSTANT", "MPU_STICK:MD_ACCEL_X_THRESHOLD_LOW:MD_ACCEL_X_THRESHOLD_LOW", "MPU_STICK:MD_ACCEL_X_THRESHOLD_HIGH:MD_ACCEL_X_THRESHOLD_HIGH", "MPU_STICK:MD_ACCEL_Y_THRESHOLD_LOW:MD_ACCEL_Y_THRESHOLD_LOW", "MPU_STICK:MD_ACCEL_Y_THRESHOLD_HIGH:MD_ACCEL_Y_THRESHOLD_HIGH", "MPU_STICK:MD_ACCEL_Z_THRESHOLD_LOW:MD_ACCEL_Z_THRESHOLD_LOW", "MPU_STICK:MD_ACCEL_Z_THRESHOLD_HIGH:MD_ACCEL_Z_THRESHOLD_HIGH", "MPU_STICK:MD_GYRO_X_THRESHOLD_LOW:MD_GYRO_X_THRESHOLD_LOW", "MPU_STICK:MD_GYRO_X_THRESHOLD_HIGH:MD_GYRO_X_THRESHOLD_HIGH", "MPU_STICK:MD_GYRO_Y_THRESHOLD_LOW:MD_GYRO_Y_THRESHOLD_LOW", "MPU_STICK:MD_GYRO_Y_THRESHOLD_HIGH:MD_GYRO_Y_THRESHOLD_HIGH", "MPU_STICK:MD_GYRO_Z_THRESHOLD_LOW:MD_GYRO_Z_THRESHOLD_LOW", "MPU_STICK:MD_GYRO_Z_THRESHOLD_HIGH:MD_GYRO_Z_THRESHOLD_HIGH", "MPU_STICK:MD_ROLL_THRESHOLD_LOW:MD_ROLL_THRESHOLD_LOW", "MPU_STICK:MD_ROLL_THRESHOLD_HIGH:MD_ROLL_THRESHOLD_HIGH", "MPU_STICK:MD_PITCH_THRESHOLD_LOW:MD_PITCH_THRESHOLD_LOW", "MPU_STICK:MD_PITCH_THRESHOLD_HIGH:MD_PITCH_THRESHOLD_HIGH", "MPU_STICK:MD_YAW_THRESHOLD_LOW:MD_YAW_THRESHOLD_LOW", "MPU_STICK:MD_YAW_THRESHOLD_HIGH:MD_YAW_THRESHOLD_HIGH", "MPU_STICK:MD_THRESHOLD_TYPE:MD_ACCEL_X_THRESHOLD_TYPE", "MPU_STICK:MD_THRESHOLD_TYPE:MD_ACCEL_Y_THRESHOLD_TYPE", "MPU_STICK:MD_THRESHOLD_TYPE:MD_ACCEL_Z_THRESHOLD_TYPE", "MPU_STICK:MD_THRESHOLD_TYPE:MD_GYRO_X_THRESHOLD_TYPE", "MPU_STICK:MD_THRESHOLD_TYPE:MD_GYRO_Y_THRESHOLD_TYPE", "MPU_STICK:MD_THRESHOLD_TYPE:MD_GYRO_Z_THRESHOLD_TYPE", "MPU_STICK:MD_THRESHOLD_TYPE:MD_ROLL_THRESHOLD_TYPE", "MPU_STICK:MD_THRESHOLD_TYPE:MD_PITCH_THRESHOLD_TYPE", "MPU_STICK:MD_THRESHOLD_TYPE:MD_YAW_THRESHOLD_TYPE"]  # MPU Stick Configuration Parameters
    n2 = case shown="Default" w8 {
      selector: w8 -> [w18 w19]
      tunnel: [w18 w19] -> _
      frame Default {
      }
      frame "IMU_ACCEL_BW" {
      }
    }
    n3 = Index Array(array=w9, index=w8) -> (element=w7:string)
    n4 = Index Array(array=w10, index=w8) -> (element=w11:string)
    n5 = case shown="\"Read All\"" w16 {
      tunnel: w15 -> [w21 w32 w402 w838 w1101]
      tunnel: [w21 w40 w420 w831 w1099] -> w14
      tunnel: w13 -> [w20 w31 w418 w836 w1097]
      tunnel: [w20 w41 w422 w827 w1100] -> w12
      tunnel: w11 -> [_ w46 _ w825 _]
      tunnel: w8 -> [_ w42 _ w837 _]
      tunnel: w10 -> [_ _ w403 _ w1098]
      tunnel: w9 -> [_ _ _ _ w1094]
      tunnel: w7 -> [_ _ _ w824 _]
      frame Default {
      }
      frame "Read" {
        n6 = Unbundle By Name(w32) -> ("Primary_references.Progress Bar"=w29:refnum<vi>)
        n7 = property class="Slide (strict)"(reference=w29, error in=w31, "Value"=u8 0, "Caption.Text"="Reading parameter") -> (error out=w30:errorcluster)  [unwired: 1 out]
        n8 = Unbundle By Name(w32) -> ("ADCP"=w56:refnum<vi>)
        n9 = property class="LVClassControl (strict)"(reference=w56) -> (reference out=w45:refnum<vi>, "Value"=w34:refnum<class "ADCP.lvclass">)  [unwired: 1 in, 1 out]
        n10 = disable-structure shown="Enabled" {
          disable-tunnel: w30 -> [w60 w61]
          disable-tunnel: [w59 w61] -> w35
          disable-tunnel: w34 -> [w58 w62]
          disable-tunnel: [w57 w62] -> w33
          frame Disabled {
            n11 = call "ADCP_Sync_Reset_Node_Connection.vi"("error in (no error)"=w60, "ADCP In"=w58) -> ("error out"=w59:errorcluster, "ADCP Out"=w57:refnum<class "ADCP.lvclass">)  [unwired: 8 in]
          }
          frame Enabled {
          }
        }
        n12 = call "ADCP_get_all_parameters.vi"("error in (no error)"=w35, "ADCP In"=w33) -> ("error out"=w55:errorcluster, "Parameters"=w54:T11, "ADCP Out"=w52:refnum<class "ADCP.lvclass">)  [unwired: 6 in, 1 out]
        n13 = for {
          tunnel: w55 -> [w399]
          tunnel: w54 -> [w396] mode=indexing
          tunnel: [w399] -> w37
          tunnel: w46 -> [w398]
          tunnel: [w396] -> w53
          tunnel: [w395] -> w38
          stop <- w395 stop-if-true
          n14 = Unbundle By Name(w396) -> ("Parameter name"=w397:string)
          n15 = Equal?(x=w398, y=w397) -> (x = y?=w395:bool)
        }
        n16 = case shown="False" w38 {
          tunnel: w37 -> [w63 w64]
          tunnel: [w63 w64] -> w36
          frame False {
          }
          frame True {
          }
        }
        n17 = Unbundle By Name(w53) -> ("Node ID"=w51:u8, "Frame ID"=w50:u8)
        n18 = Build Array(w50) -> (w49:u8[])
        n19 = call "ADCP_Remote_Request_Frames.vi"("error in (no error)"=w36, "Request Frame IDs"=w49, "Node ID"=w51, "ADCP In"=w52) -> ("error out"=w47:errorcluster, "ADCP Out"=w48:refnum<class "ADCP.lvclass">)  [unwired: 4 in, 2 out]
        n20 = call "ADCP_read_parameter.vi"("error in (no error)"=w47, "Parameter Name"=w46, "ADCP In"=w48) -> ("error out"=w26:errorcluster, "Parameter Value"=w39:string, "ADCP out"=w44:refnum<class "ADCP.lvclass">)  [unwired: 5 in, 1 out]
        "Parameter Value" <- w39
        n21 = property class="LVClassControl (strict)"(reference=w45, "Value"=w44) -> (reference out=w43:refnum<vi>)  [unwired: 1 in, 1 out]
        n22 = Bundle By Name(cluster=w32, "ADCP"=w43) -> (w23:T1)
        n23 = Unbundle By Name(w23) -> ("Primary_references.Progress Bar"=w22:refnum<vi>)
        n24 = property class="Slide (strict)"(reference=w22, error in=w26, "Value"=u8 100) -> (error out=w25:errorcluster)  [unwired: 1 out]
        n25 = case shown="\"MP_DETECTION_TYPE_X_ACCEL\"" w42 {
          tunnel: w25 -> [w66 w71 w80 w90 w99 w109 w117 w125 w134 w143 w152 w160 w168 w176 w184 w192 w200 w208 w216 w224 w232 w240 w248 w256 w264 w272 w280 w288 w296 w304 w312 w321 w330 w339 w348 w357 w366 w375 w384 w393]
          tunnel: [w66 w70 w79 w89 w98 w108 w116 w124 w133 w142 w151 w159 w167 w175 w183 w191 w199 w207 w215 w223 w231 w239 w247 w255 w263 w271 w279 w287 w295 w303 w311 w320 w329 w338 w347 w356 w365 w374 w383 w392] -> w41
          tunnel: w23 -> [w65 w69 w78 w88 w97 w107 w115 w123 w132 w141 w150 w158 w166 w174 w182 w190 w198 w206 w214 w222 w230 w238 w246 w254 w262 w270 w278 w286 w294 w302 w310 w319 w328 w337 w346 w355 w364 w373 w382 w391]
          tunnel: [w65 w67 w76 w86 w95 w105 w113 w121 w130 w139 w148 w156 w164 w172 w180 w188 w196 w204 w212 w220 w228 w236 w244 w252 w260 w268 w276 w284 w292 w300 w308 w317 w326 w335 w344 w353 w362 w371 w380 w389] -> w40
          tunnel: w39 -> [_ w75 w84 w93 w102 w104 w112 w120 w128 w137 w146 w155 w163 w171 w179 w187 w195 w203 w211 w219 w227 w235 w243 w251 w259 w267 w275 w283 w291 w299 w307 w316 w325 w334 w343 w352 w361 w370 w379 w388]
          frame Default {
          }
          frame "IMU_ACCEL_FS" {
            n26 = Unbundle By Name(w69) -> ("IMU_configuration_references.IMU Accelerometer F.S. value"=w73:refnum<vi>)
            n27 = Search 1D Array(1D array=string[] ["IMU_ACCEL_FS_2G", "IMU_ACCEL_FS_4G", "IMU_ACCEL_FS_8G", "IMU_ACCEL_FS_16G"], element=w75) -> (index of element=w72:i32)  [unwired: 1 in]
            n28 = property class="Enum (strict)"(reference=w73, error in=w71, "Value"=w72) -> (reference out=w68:refnum<vi>, error out=w70:errorcluster)
            n29 = Bundle By Name(cluster=w69, "IMU_configuration_references.IMU Accelerometer F.S. value"=w68) -> (w67:T1)
          }
          frame "IMU_ACCEL_BW" {
            # "IMU_ACCEL_BW_460Hz:IMU_ACCEL_BW_184Hz:IMU_ACCEL_BW_92Hz:IMU_ACCEL_BW_41Hz:IMU_ACCEL_BW_20Hz:IMU_ACCEL_BW_10Hz:IMU_ACCEL_BW_5Hz"
            n30 = Unbundle By Name(w78) -> ("IMU_configuration_references.IMU Accelerometer bandwidth"=w82:refnum<vi>)
            n31 = Search 1D Array(1D array=string[] ["IMU_ACCEL_BW_460Hz", "IMU_ACCEL_BW_184Hz", "IMU_ACCEL_BW_92Hz", "IMU_ACCEL_BW_41Hz", "IMU_ACCEL_BW_20Hz", "IMU_ACCEL_BW_10Hz", "IMU_ACCEL_BW_5Hz"], element=w84) -> (index of element=w81:i32)  [unwired: 1 in]
            n32 = property class="Enum (strict)"(reference=w82, error in=w80, "Value"=w81) -> (reference out=w77:refnum<vi>, error out=w79:errorcluster)
            n33 = Bundle By Name(cluster=w78, "IMU_configuration_references.IMU Accelerometer bandwidth"=w77) -> (w76:T1)
          }
          frame "IMU_GYRO_FS" {
            # "IMU_GYRO_FS_250DPS:IMU_GYRO_FS_500DPS:IMU_GYRO_FS_1000DPS:IMU_GYRO_FS_2000DPS"
            n34 = Unbundle By Name(w88) -> ("IMU_configuration_references.IMU Gyroscope F.S. value"=w92:refnum<vi>)
            n35 = Search 1D Array(1D array=string[] ["IMU_GYRO_FS_250DPS", "IMU_GYRO_FS_500DPS", "IMU_GYRO_FS_1000DPS", "IMU_GYRO_FS_2000DPS"], element=w93) -> (index of element=w91:i32)  [unwired: 1 in]
            n36 = property class="Enum (strict)"(reference=w92, error in=w90, "Value"=w91) -> (reference out=w87:refnum<vi>, error out=w89:errorcluster)
            n37 = Bundle By Name(cluster=w88, "IMU_configuration_references.IMU Gyroscope F.S. value"=w87) -> (w86:T1)
          }
          frame "IMU_GYRO_BW" {
            # "IMU_GYRO_BW_NONE:IMU_GYRO_BW_184Hz:IMU_GYRO_BW_92Hz:IMU_GYRO_BW_41Hz:IMU_GYRO_BW_20Hz:IMU_GYRO_BW_10Hz:IMU_GYRO_BW_5Hz"
            n38 = Unbundle By Name(w97) -> ("IMU_configuration_references.IMU Gyroscope bandwidth"=w101:refnum<vi>)
            n39 = Search 1D Array(1D array=string[] ["IMU_GYRO_BW_NONE", "IMU_GYRO_BW_184Hz", "IMU_GYRO_BW_92Hz", "IMU_GYRO_BW_41Hz", "IMU_GYRO_BW_20Hz", "IMU_GYRO_BW_10Hz", "IMU_GYRO_BW_5Hz"], element=w102) -> (index of element=w100:i32)  [unwired: 1 in]
            n40 = property class="Enum (strict)"(reference=w101, error in=w99, "Value"=w100) -> (reference out=w96:refnum<vi>, error out=w98:errorcluster)
            n41 = Bundle By Name(cluster=w97, "IMU_configuration_references.IMU Gyroscope bandwidth"=w96) -> (w95:T1)
          }
          frame "IMU_CALIB_INTERVAL" {
            n42 = Unbundle By Name(w107) -> ("IMU_configuration_references.Calibration interval (ms)"=w110:refnum<vi>)
            n43 = Decimal String To Number(string=w104) -> (number=w103:i32)  [unwired: 2 in, 1 out]
            n44 = property class="DigNum (strict)"(reference=w110, error in=w109, "Value"=w103) -> (reference out=w106:refnum<vi>, error out=w108:errorcluster)
            n45 = Bundle By Name(cluster=w107, "IMU_configuration_references.Calibration interval (ms)"=w106) -> (w105:T1)
          }
          frame "IMU_CALIB_POINT_COUNT" {
            n46 = Unbundle By Name(w115) -> ("IMU_configuration_references.Calibration point count"=w118:refnum<vi>)
            n47 = Decimal String To Number(string=w112) -> (number=w111:i32)  [unwired: 2 in, 1 out]
            n48 = property class="DigNum (strict)"(reference=w118, error in=w117, "Value"=w111) -> (reference out=w114:refnum<vi>, error out=w116:errorcluster)
            n49 = Bundle By Name(cluster=w115, "IMU_configuration_references.Calibration point count"=w114) -> (w113:T1)
          }
          frame "IMU_SAMPLING_FREQ" {
            n50 = Unbundle By Name(w123) -> ("IMU_configuration_references.Sampling frequency (Hz)"=w126:refnum<vi>)
            n51 = Decimal String To Number(string=w120) -> (number=w119:i32)  [unwired: 2 in, 1 out]
            n52 = property class="DigNum (strict)"(reference=w126, error in=w125, "Value"=w119) -> (reference out=w122:refnum<vi>, error out=w124:errorcluster)
            n53 = Bundle By Name(cluster=w123, "IMU_configuration_references.Sampling frequency (Hz)"=w122) -> (w121:T1)
          }
          frame "LED1_CONFIG" {
            n54 = Unbundle By Name(w132) -> ("LED_Configuration_References.LED1 Configuration"=w135:refnum<vi>)
            n55 = Search 1D Array(1D array=string[] ["USER_CONTROLLED_DIG_OUTPUT", "X_ACCEL_PWM", "Y_ACCEL_PWM", "Z_ACCEL_PWM", "X_ACCEL_MD_OUTPUT", "Y_ACCEL_MD_OUTPUT", "Z_ACCEL_MD_OUTPUT", "X_GYRO_PWM", "Y_ACCEL_PWM", "Z_ACCEL_PWM", "X_GYRO_MD_OUTPUT", "Y_GYRO_MD_OUTPUT", "Z_GYRO_MD_OUTPUT", "ROLL_PWM", "PITCH_PWM", "YAW_PWM", "ROLL_MD_OUTPUT", "PITCH_MD_OUTPUT", "YAW_MD_OUTPUT", "USER_CONTROLLED_PWM_OUTPUT"] ("Array"), element=w128) -> (index of element=w127:i32)  [unwired: 1 in]
            n56 = property class="Enum (strict)"(reference=w135, error in=w134, "Value"=w127) -> (reference out=w131:refnum<vi>, error out=w133:errorcluster)
            n57 = Bundle By Name(cluster=w132, "LED_Configuration_References.LED1 Configuration"=w131) -> (w130:T1)
          }
          frame "LED2_CONFIG" {
            n58 = Unbundle By Name(w141) -> ("LED_Configuration_References.LED2 Configuration"=w144:refnum<vi>)
            n59 = Search 1D Array(1D array=string[] ["USER_CONTROLLED_DIG_OUTPUT", "X_ACCEL_PWM", "Y_ACCEL_PWM", "Z_ACCEL_PWM", "X_ACCEL_MD_OUTPUT", "Y_ACCEL_MD_OUTPUT", "Z_ACCEL_MD_OUTPUT", "X_GYRO_PWM", "Y_ACCEL_PWM", "Z_ACCEL_PWM", "X_GYRO_MD_OUTPUT", "Y_GYRO_MD_OUTPUT", "Z_GYRO_MD_OUTPUT", "ROLL_PWM", "PITCH_PWM", "YAW_PWM", "ROLL_MD_OUTPUT", "PITCH_MD_OUTPUT", "YAW_MD_OUTPUT", "USER_CONTROLLED_PWM_OUTPUT"] ("Array"), element=w137) -> (index of element=w136:i32)  [unwired: 1 in]
            n60 = property class="Enum (strict)"(reference=w144, error in=w143, "Value"=w136) -> (reference out=w140:refnum<vi>, error out=w142:errorcluster)
            n61 = Bundle By Name(cluster=w141, "LED_Configuration_References.LED2 Configuration"=w140) -> (w139:T1)
          }
          frame "LED3_CONFIG" {
            n62 = Unbundle By Name(w150) -> ("LED_Configuration_References.LED3 Configuration"=w153:refnum<vi>)
            n63 = Search 1D Array(1D array=string[] ["USER_CONTROLLED_DIG_OUTPUT", "X_ACCEL_PWM", "Y_ACCEL_PWM", "Z_ACCEL_PWM", "X_ACCEL_MD_OUTPUT", "Y_ACCEL_MD_OUTPUT", "Z_ACCEL_MD_OUTPUT", "X_GYRO_PWM", "Y_ACCEL_PWM", "Z_ACCEL_PWM", "X_GYRO_MD_OUTPUT", "Y_GYRO_MD_OUTPUT", "Z_GYRO_MD_OUTPUT", "ROLL_PWM", "PITCH_PWM", "YAW_PWM", "ROLL_MD_OUTPUT", "PITCH_MD_OUTPUT", "YAW_MD_OUTPUT", "USER_CONTROLLED_PWM_OUTPUT"] ("Array"), element=w146) -> (index of element=w145:i32)  [unwired: 1 in]
            n64 = property class="Enum (strict)"(reference=w153, error in=w152, "Value"=w145) -> (reference out=w149:refnum<vi>, error out=w151:errorcluster)
            n65 = Bundle By Name(cluster=w150, "LED_Configuration_References.LED3 Configuration"=w149) -> (w148:T1)
          }
          frame "MP_ROLL_FILTER_CONSTANT" {
            n66 = Unbundle By Name(w158) -> ("MP_Comp_Filter_Constants_References.Roll filter constant"=w161:refnum<vi>)
            n67 = Fract/Exp String To Number(string=w155) -> (number=w154:dbl)  [unwired: 3 in, 1 out]
            n68 = property class="DigNum (strict)"(reference=w161, error in=w160, "Value"=w154) -> (reference out=w157:refnum<vi>, error out=w159:errorcluster)
            n69 = Bundle By Name(cluster=w158, "MP_Comp_Filter_Constants_References.Roll filter constant"=w157) -> (w156:T1)
          }
          frame "MP_PITCH_FILTER_CONSTANT" {
            n70 = Unbundle By Name(w166) -> ("MP_Comp_Filter_Constants_References.Pitch filter constant"=w169:refnum<vi>)
            n71 = Fract/Exp String To Number(string=w163) -> (number=w162:dbl)  [unwired: 3 in, 1 out]
            n72 = property class="DigNum (strict)"(reference=w169, error in=w168, "Value"=w162) -> (reference out=w165:refnum<vi>, error out=w167:errorcluster)
            n73 = Bundle By Name(cluster=w166, "MP_Comp_Filter_Constants_References.Pitch filter constant"=w165) -> (w164:T1)
          }
          frame "MP_THRESHOLD_X_ACCEL_LOW" {
            n74 = Unbundle By Name(w174) -> ("MD_Threshold_References.X accel. threshold (L)"=w177:refnum<vi>)
            n75 = Fract/Exp String To Number(string=w171) -> (number=w170:dbl)  [unwired: 3 in, 1 out]
            n76 = property class="DigNum (strict)"(reference=w177, error in=w176, "Value"=w170) -> (reference out=w173:refnum<vi>, error out=w175:errorcluster)
            n77 = Bundle By Name(cluster=w174, "MD_Threshold_References.X accel. threshold (L)"=w173) -> (w172:T1)
          }
          frame "MP_THRESHOLD_X_ACCEL_HIGH" {
            n78 = Unbundle By Name(w182) -> ("MD_Threshold_References.X accel. threshold (U)"=w185:refnum<vi>)
            n79 = Fract/Exp String To Number(string=w179) -> (number=w178:dbl)  [unwired: 3 in, 1 out]
            n80 = property class="DigNum (strict)"(reference=w185, error in=w184, "Value"=w178) -> (reference out=w181:refnum<vi>, error out=w183:errorcluster)
            n81 = Bundle By Name(cluster=w182, "MD_Threshold_References.X accel. threshold (U)"=w181) -> (w180:T1)
          }
          frame "MP_THRESHOLD_Y_ACCEL_LOW" {
            n82 = Unbundle By Name(w190) -> ("MD_Threshold_References.Y accel. threshold (L)"=w193:refnum<vi>)
            n83 = Fract/Exp String To Number(string=w187) -> (number=w186:dbl)  [unwired: 3 in, 1 out]
            n84 = property class="DigNum (strict)"(reference=w193, error in=w192, "Value"=w186) -> (reference out=w189:refnum<vi>, error out=w191:errorcluster)
            n85 = Bundle By Name(cluster=w190, "MD_Threshold_References.Y accel. threshold (L)"=w189) -> (w188:T1)
          }
          frame "MP_THRESHOLD_Y_ACCEL_HIGH" {
            n86 = Unbundle By Name(w198) -> ("MD_Threshold_References.Y accel. threshold (U)"=w201:refnum<vi>)
            n87 = Fract/Exp String To Number(string=w195) -> (number=w194:dbl)  [unwired: 3 in, 1 out]
            n88 = property class="DigNum (strict)"(reference=w201, error in=w200, "Value"=w194) -> (reference out=w197:refnum<vi>, error out=w199:errorcluster)
            n89 = Bundle By Name(cluster=w198, "MD_Threshold_References.Y accel. threshold (U)"=w197) -> (w196:T1)
          }
          frame "MP_THRESHOLD_Z_ACCEL_LOW" {
            n90 = Unbundle By Name(w206) -> ("MD_Threshold_References.Z accel. threshold (L)"=w209:refnum<vi>)
            n91 = Fract/Exp String To Number(string=w203) -> (number=w202:dbl)  [unwired: 3 in, 1 out]
            n92 = property class="DigNum (strict)"(reference=w209, error in=w208, "Value"=w202) -> (reference out=w205:refnum<vi>, error out=w207:errorcluster)
            n93 = Bundle By Name(cluster=w206, "MD_Threshold_References.Z accel. threshold (L)"=w205) -> (w204:T1)
          }
          frame "MP_THRESHOLD_Z_ACCEL_HIGH" {
            n94 = Unbundle By Name(w214) -> ("MD_Threshold_References.Z accel. threshold (U)"=w217:refnum<vi>)
            n95 = Fract/Exp String To Number(string=w211) -> (number=w210:dbl)  [unwired: 3 in, 1 out]
            n96 = property class="DigNum (strict)"(reference=w217, error in=w216, "Value"=w210) -> (reference out=w213:refnum<vi>, error out=w215:errorcluster)
            n97 = Bundle By Name(cluster=w214, "MD_Threshold_References.Z accel. threshold (U)"=w213) -> (w212:T1)
          }
          frame "MP_THRESHOLD_X_GYRO_LOW" {
            n98 = Unbundle By Name(w222) -> ("MD_Threshold_References.X gyro. threshold (L)"=w225:refnum<vi>)
            n99 = Fract/Exp String To Number(string=w219) -> (number=w218:dbl)  [unwired: 3 in, 1 out]
            n100 = property class="DigNum (strict)"(reference=w225, error in=w224, "Value"=w218) -> (reference out=w221:refnum<vi>, error out=w223:errorcluster)
            n101 = Bundle By Name(cluster=w222, "MD_Threshold_References.X gyro. threshold (L)"=w221) -> (w220:T1)
          }
          frame "MP_THRESHOLD_X_GYRO_HIGH" {
            n102 = Unbundle By Name(w230) -> ("MD_Threshold_References.X gyro. threshold (U)"=w233:refnum<vi>)
            n103 = Fract/Exp String To Number(string=w227) -> (number=w226:dbl)  [unwired: 3 in, 1 out]
            n104 = property class="DigNum (strict)"(reference=w233, error in=w232, "Value"=w226) -> (reference out=w229:refnum<vi>, error out=w231:errorcluster)
            n105 = Bundle By Name(cluster=w230, "MD_Threshold_References.X gyro. threshold (U)"=w229) -> (w228:T1)
          }
          frame "MP_THRESHOLD_Y_GYRO_LOW" {
            n106 = Unbundle By Name(w238) -> ("MD_Threshold_References.Y gyro. threshold (L)"=w241:refnum<vi>)
            n107 = Fract/Exp String To Number(string=w235) -> (number=w234:dbl)  [unwired: 3 in, 1 out]
            n108 = property class="DigNum (strict)"(reference=w241, error in=w240, "Value"=w234) -> (reference out=w237:refnum<vi>, error out=w239:errorcluster)
            n109 = Bundle By Name(cluster=w238, "MD_Threshold_References.Y gyro. threshold (L)"=w237) -> (w236:T1)
          }
          frame "MP_THRESHOLD_Y_GYRO_HIGH" {
            n110 = Unbundle By Name(w246) -> ("MD_Threshold_References.Y gyro. threshold (U)"=w249:refnum<vi>)
            n111 = Fract/Exp String To Number(string=w243) -> (number=w242:dbl)  [unwired: 3 in, 1 out]
            n112 = property class="DigNum (strict)"(reference=w249, error in=w248, "Value"=w242) -> (reference out=w245:refnum<vi>, error out=w247:errorcluster)
            n113 = Bundle By Name(cluster=w246, "MD_Threshold_References.Y gyro. threshold (U)"=w245) -> (w244:T1)
          }
          frame "MP_THRESHOLD_Z_GYRO_LOW" {
            n114 = Unbundle By Name(w254) -> ("MD_Threshold_References.Z gyro. threshold (L)"=w257:refnum<vi>)
            n115 = Fract/Exp String To Number(string=w251) -> (number=w250:dbl)  [unwired: 3 in, 1 out]
            n116 = property class="DigNum (strict)"(reference=w257, error in=w256, "Value"=w250) -> (reference out=w253:refnum<vi>, error out=w255:errorcluster)
            n117 = Bundle By Name(cluster=w254, "MD_Threshold_References.Z gyro. threshold (L)"=w253) -> (w252:T1)
          }
          frame "MP_THRESHOLD_Z_GYRO_HIGH" {
            n118 = Unbundle By Name(w262) -> ("MD_Threshold_References.Z gyro. threshold (U)"=w265:refnum<vi>)
            n119 = Fract/Exp String To Number(string=w259) -> (number=w258:dbl)  [unwired: 3 in, 1 out]
            n120 = property class="DigNum (strict)"(reference=w265, error in=w264, "Value"=w258) -> (reference out=w261:refnum<vi>, error out=w263:errorcluster)
            n121 = Bundle By Name(cluster=w262, "MD_Threshold_References.Z gyro. threshold (U)"=w261) -> (w260:T1)
          }
          frame "MP_THRESHOLD_ROLL_LOW" {
            n122 = Unbundle By Name(w270) -> ("MD_Threshold_References.Roll threshold (L)"=w273:refnum<vi>)
            n123 = Fract/Exp String To Number(string=w267) -> (number=w266:dbl)  [unwired: 3 in, 1 out]
            n124 = property class="DigNum (strict)"(reference=w273, error in=w272, "Value"=w266) -> (reference out=w269:refnum<vi>, error out=w271:errorcluster)
            n125 = Bundle By Name(cluster=w270, "MD_Threshold_References.Roll threshold (L)"=w269) -> (w268:T1)
          }
          frame "MP_THRESHOLD_ROLL_HIGH" {
            n126 = Unbundle By Name(w278) -> ("MD_Threshold_References.Roll threshold (U)"=w281:refnum<vi>)
            n127 = Fract/Exp String To Number(string=w275) -> (number=w274:dbl)  [unwired: 3 in, 1 out]
            n128 = property class="DigNum (strict)"(reference=w281, error in=w280, "Value"=w274) -> (reference out=w277:refnum<vi>, error out=w279:errorcluster)
            n129 = Bundle By Name(cluster=w278, "MD_Threshold_References.Roll threshold (U)"=w277) -> (w276:T1)
          }
          frame "MP_THRESHOLD_PITCH_LOW" {
            n130 = Unbundle By Name(w286) -> ("MD_Threshold_References.Pitch. threshold (L)"=w289:refnum<vi>)
            n131 = Fract/Exp String To Number(string=w283) -> (number=w282:dbl)  [unwired: 3 in, 1 out]
            n132 = property class="DigNum (strict)"(reference=w289, error in=w288, "Value"=w282) -> (reference out=w285:refnum<vi>, error out=w287:errorcluster)
            n133 = Bundle By Name(cluster=w286, "MD_Threshold_References.Pitch. threshold (L)"=w285) -> (w284:T1)
          }
          frame "MP_THRESHOLD_PITCH_HIGH" {
            n134 = Unbundle By Name(w294) -> ("MD_Threshold_References.Pitch threshold (U)"=w297:refnum<vi>)
            n135 = Fract/Exp String To Number(string=w291) -> (number=w290:dbl)  [unwired: 3 in, 1 out]
            n136 = property class="DigNum (strict)"(reference=w297, error in=w296, "Value"=w290) -> (reference out=w293:refnum<vi>, error out=w295:errorcluster)
            n137 = Bundle By Name(cluster=w294, "MD_Threshold_References.Pitch threshold (U)"=w293) -> (w292:T1)
          }
          frame "MP_THRESHOLD_YAW_LOW" {
            n138 = Unbundle By Name(w302) -> ("MD_Threshold_References.Yaw threshold (L)"=w305:refnum<vi>)
            n139 = Fract/Exp String To Number(string=w299) -> (number=w298:dbl)  [unwired: 3 in, 1 out]
            n140 = property class="DigNum (strict)"(reference=w305, error in=w304, "Value"=w298) -> (reference out=w301:refnum<vi>, error out=w303:errorcluster)
            n141 = Bundle By Name(cluster=w302, "MD_Threshold_References.Yaw threshold (L)"=w301) -> (w300:T1)
          }
          frame "MP_THRESHOLD_YAW_HIGH" {
            n142 = Unbundle By Name(w310) -> ("MD_Threshold_References.Yaw threshold (U)"=w313:refnum<vi>)
            n143 = Fract/Exp String To Number(string=w307) -> (number=w306:dbl)  [unwired: 3 in, 1 out]
            n144 = property class="DigNum (strict)"(reference=w313, error in=w312, "Value"=w306) -> (reference out=w309:refnum<vi>, error out=w311:errorcluster)
            n145 = Bundle By Name(cluster=w310, "MD_Threshold_References.Yaw threshold (U)"=w309) -> (w308:T1)
          }
          frame "MP_DETECTION_TYPE_X_ACCEL" {
            n146 = Unbundle By Name(w319) -> ("MD_Type_References.X accel threshold type"=w322:refnum<vi>)
            n147 = Search 1D Array(1D array=string[] ["ABS_LESSER_THAN", "ABS_GREATER_THAN", "LESSER_THAN", "GREATER_THAN", "WINDOWED_MODE_WITHIN_BOUNDS", "WINDOWED_MODE_OUTSIDE_BOUNDS"] ("Array"), element=w316) -> (index of element=w315:i32)  [unwired: 1 in]
            n148 = property class="Enum (strict)"(reference=w322, error in=w321, "Value"=w315) -> (reference out=w318:refnum<vi>, error out=w320:errorcluster)
            n149 = Bundle By Name(cluster=w319, "MD_Type_References.X accel threshold type"=w318) -> (w317:T1)
          }
          frame "MP_DETECTION_TYPE_Y_ACCEL" {
            n150 = Unbundle By Name(w328) -> ("MD_Type_References.Y accel threshold type"=w331:refnum<vi>)
            n151 = Search 1D Array(1D array=string[] ["ABS_LESSER_THAN", "ABS_GREATER_THAN", "LESSER_THAN", "GREATER_THAN", "WINDOWED_MODE_WITHIN_BOUNDS", "WINDOWED_MODE_OUTSIDE_BOUNDS"] ("Array"), element=w325) -> (index of element=w324:i32)  [unwired: 1 in]
            n152 = property class="Enum (strict)"(reference=w331, error in=w330, "Value"=w324) -> (reference out=w327:refnum<vi>, error out=w329:errorcluster)
            n153 = Bundle By Name(cluster=w328, "MD_Type_References.Y accel threshold type"=w327) -> (w326:T1)
          }
          frame "MP_DETECTION_TYPE_Z_ACCEL" {
            n154 = Unbundle By Name(w337) -> ("MD_Type_References.Z accel threshold type"=w340:refnum<vi>)
            n155 = Search 1D Array(1D array=string[] ["ABS_LESSER_THAN", "ABS_GREATER_THAN", "LESSER_THAN", "GREATER_THAN", "WINDOWED_MODE_WITHIN_BOUNDS", "WINDOWED_MODE_OUTSIDE_BOUNDS"] ("Array"), element=w334) -> (index of element=w333:i32)  [unwired: 1 in]
            n156 = property class="Enum (strict)"(reference=w340, error in=w339, "Value"=w333) -> (reference out=w336:refnum<vi>, error out=w338:errorcluster)
            n157 = Bundle By Name(cluster=w337, "MD_Type_References.Z accel threshold type"=w336) -> (w335:T1)
          }
          frame "MP_DETECTION_TYPE_X_GYRO" {
            n158 = Unbundle By Name(w346) -> ("MD_Type_References.X gyro threshold type"=w349:refnum<vi>)
            n159 = Search 1D Array(1D array=string[] ["ABS_LESSER_THAN", "ABS_GREATER_THAN", "LESSER_THAN", "GREATER_THAN", "WINDOWED_MODE_WITHIN_BOUNDS", "WINDOWED_MODE_OUTSIDE_BOUNDS"] ("Array"), element=w343) -> (index of element=w342:i32)  [unwired: 1 in]
            n160 = property class="Enum (strict)"(reference=w349, error in=w348, "Value"=w342) -> (reference out=w345:refnum<vi>, error out=w347:errorcluster)
            n161 = Bundle By Name(cluster=w346, "MD_Type_References.X gyro threshold type"=w345) -> (w344:T1)
          }
          frame "MP_DETECTION_TYPE_Y_GYRO" {
            n162 = Unbundle By Name(w355) -> ("MD_Type_References.Y gyro threshold type"=w358:refnum<vi>)
            n163 = Search 1D Array(1D array=string[] ["ABS_LESSER_THAN", "ABS_GREATER_THAN", "LESSER_THAN", "GREATER_THAN", "WINDOWED_MODE_WITHIN_BOUNDS", "WINDOWED_MODE_OUTSIDE_BOUNDS"] ("Array"), element=w352) -> (index of element=w351:i32)  [unwired: 1 in]
            n164 = property class="Enum (strict)"(reference=w358, error in=w357, "Value"=w351) -> (reference out=w354:refnum<vi>, error out=w356:errorcluster)
            n165 = Bundle By Name(cluster=w355, "MD_Type_References.Y gyro threshold type"=w354) -> (w353:T1)
          }
          frame "MP_DETECTION_TYPE_Z_GYRO" {
            n166 = Unbundle By Name(w364) -> ("MD_Type_References.Z gyro threshold type"=w367:refnum<vi>)
            n167 = Search 1D Array(1D array=string[] ["ABS_LESSER_THAN", "ABS_GREATER_THAN", "LESSER_THAN", "GREATER_THAN", "WINDOWED_MODE_WITHIN_BOUNDS", "WINDOWED_MODE_OUTSIDE_BOUNDS"] ("Array"), element=w361) -> (index of element=w360:i32)  [unwired: 1 in]
            n168 = property class="Enum (strict)"(reference=w367, error in=w366, "Value"=w360) -> (reference out=w363:refnum<vi>, error out=w365:errorcluster)
            n169 = Bundle By Name(cluster=w364, "MD_Type_References.Z gyro threshold type"=w363) -> (w362:T1)
          }
          frame "MP_DETECTION_TYPE_ROLL" {
            n170 = Unbundle By Name(w373) -> ("MD_Type_References.Roll threshold type"=w376:refnum<vi>)
            n171 = Search 1D Array(1D array=string[] ["ABS_LESSER_THAN", "ABS_GREATER_THAN", "LESSER_THAN", "GREATER_THAN", "WINDOWED_MODE_WITHIN_BOUNDS", "WINDOWED_MODE_OUTSIDE_BOUNDS"] ("Array"), element=w370) -> (index of element=w369:i32)  [unwired: 1 in]
            n172 = property class="Enum (strict)"(reference=w376, error in=w375, "Value"=w369) -> (reference out=w372:refnum<vi>, error out=w374:errorcluster)
            n173 = Bundle By Name(cluster=w373, "MD_Type_References.Roll threshold type"=w372) -> (w371:T1)
          }
          frame "MP_DETECTION_TYPE_PITCH" {
            n174 = Unbundle By Name(w382) -> ("MD_Type_References.Pitch threshold type"=w385:refnum<vi>)
            n175 = Search 1D Array(1D array=string[] ["ABS_LESSER_THAN", "ABS_GREATER_THAN", "LESSER_THAN", "GREATER_THAN", "WINDOWED_MODE_WITHIN_BOUNDS", "WINDOWED_MODE_OUTSIDE_BOUNDS"] ("Array"), element=w379) -> (index of element=w378:i32)  [unwired: 1 in]
            n176 = property class="Enum (strict)"(reference=w385, error in=w384, "Value"=w378) -> (reference out=w381:refnum<vi>, error out=w383:errorcluster)
            n177 = Bundle By Name(cluster=w382, "MD_Type_References.Pitch threshold type"=w381) -> (w380:T1)
          }
          frame "MP_DETECTION_TYPE_YAW" {
            n178 = Unbundle By Name(w391) -> ("MD_Type_References.Yaw threshold type"=w394:refnum<vi>)
            n179 = Search 1D Array(1D array=string[] ["ABS_LESSER_THAN", "ABS_GREATER_THAN", "LESSER_THAN", "GREATER_THAN", "WINDOWED_MODE_WITHIN_BOUNDS", "WINDOWED_MODE_OUTSIDE_BOUNDS"] ("Array"), element=w388) -> (index of element=w387:i32)  [unwired: 1 in]
            n180 = property class="Enum (strict)"(reference=w394, error in=w393, "Value"=w387) -> (reference out=w390:refnum<vi>, error out=w392:errorcluster)
            n181 = Bundle By Name(cluster=w391, "MD_Type_References.Yaw threshold type"=w390) -> (w389:T1)
          }
        }
      }
      frame "Read All" {
        n182 = Unbundle By Name(w402) -> ("Primary_references.Progress Bar"=w400:refnum<vi>)
        n183 = Unbundle By Name(w402) -> ("ADCP"=w427:refnum<vi>)
        n184 = property class="LVClassControl (strict)"(reference=w427) -> (reference out=w426:refnum<vi>, "Value"=w417:refnum<class "ADCP.lvclass">)  [unwired: 1 in, 1 out]
        n185 = Array Size(array=w403) -> ()  [unwired: 1 out]
        n186 = for {
          tunnel: w403 -> [w812] mode=indexing
          shift-right: [w811] -> w406
          shift-left: w417 -> [w816]
          shift-right: [w810] -> w416
          shift-left: w418 -> [w817]
          tunnel: [w808] -> w415 mode=indexing
          n187 = call "ADCP_get_all_parameters.vi"("error in (no error)"=w817, "ADCP In"=w816) -> ("error out"=w815:errorcluster, "Parameters"=w813:T11, "ADCP Out"=w814:refnum<class "ADCP.lvclass">)  [unwired: 6 in, 1 out]
          n188 = for {
            shift-right: [w820] -> w810
            shift-left: w815 -> [w820]
            shift-right: [w821] -> w811
            shift-left: w814 -> [w821]
            tunnel: w813 -> [w818] mode=indexing
            tunnel: w812 -> [w822]
            tunnel: [w818] -> w809
            stop <- w819 stop-if-true
            n189 = Unbundle By Name(w818) -> ("Parameter name"=w823:string)
            n190 = Equal?(x=w822, y=w823) -> (x = y?=w819:bool)
          }
          n191 = Unbundle By Name(w809) -> ("Frame ID"=w808:u8)
        }
        n192 = for {
          tunnel: w415 -> [w804] mode=indexing
          shift-right: [w806] -> _
          shift-left: -1 -> [w807]
          shift-right: [w805] -> w407
          shift-left: w416 -> [w805]
          tunnel: [w804] -> w408 mode=indexing if=w803
          n193 = Not Equal?(x=w804, y=w807) -> (x != y?=w803:bool)
          n194 = Select(t=w804, s=w803, f=w807) -> (s? t:f=w806:i32)
        }
        n195 = Array Size(array=w408) -> (size(s)=w413:i32)
        n196 = To Double Precision Float(number=w413) -> (double precision float=w412:dbl)
        n197 = Divide(x=w412, y=4.0) -> (x/y=w410:dbl)
        n198 = To Unsigned Long Integer(number=w410) -> (unsigned 32bit integer=w409:u32)
        n199 = Increment(x=w409) -> (x+1=w401:u32)
        n200 = for {
          N: w401 -> [_]
          tunnel: w408 -> [w791]
          shift-right: [w773] -> w405
          shift-left: w407 -> [w794]
          shift-right: [w792] -> w404
          shift-left: w406 -> [w793]
          tunnel: w401 -> [w777]
          tunnel: w400 -> [w775]
          i -> [w776]
          w789 = 4 ("x")
          n201 = Increment(x=w776) -> (x+1=w783:i32)
          n202 = Multiply(x=w789, y=w776) -> (x*y=w790:i32)
          n203 = To Double Precision Float(number=w783) -> (double precision float=w785:dbl)
          n204 = To Double Precision Float(number=w777) -> (double precision float=w784:dbl)
          n205 = Array Subset(array=w791, index=w790, length=w789) -> (w788:u8[])
          n206 = Divide(x=w785, y=w784) -> (x/y=w782:dbl)
          n207 = Multiply(x=w782, y=100.0) -> (x*y=w780:dbl)
          n208 = To Unsigned Byte Integer(number=w780) -> (unsigned 8bit integer=w779:u8)
          n209 = Array Size(array=w788) -> (size(s)=w787:i32)
          n210 = Not Equal To 0?(x=w787) -> (x != 0?=w786:bool)
          n211 = property class="Slide (strict)"(reference=w775, "Value"=w779, "Caption.Text"="Reading all configurations") -> ()  [unwired: 1 in, 2 out]
          n212 = case shown="True" w786 {
            tunnel: w794 -> [w796 w802]
            tunnel: w793 -> [w795 w800]
            tunnel: [w795 w799] -> w792
            tunnel: [w796 w798] -> w774
            tunnel: w788 -> [_ w797]
            frame False {
            }
            frame True {
              n213 = call "ADCP_Remote_Request_Frames.vi"("error in (no error)"=w802, "Request Frame IDs"=w797, "Node ID"=0, "ADCP In"=w800) -> ("error out"=w798:errorcluster, "ADCP Out"=w799:refnum<class "ADCP.lvclass">)  [unwired: 4 in, 2 out]
            }
          }
          n214 = call <vilib>:"Clear Errors.vi"("error in (no error)"=w774) -> ("error out"=w773:errorcluster)  [unwired: 5 in, 1 out]
        }
        n215 = for {
          tunnel: [w770] -> w419 mode=indexing
          shift-right: [w771] -> w423
          shift-left: w405 -> [w769]
          shift-right: [w772] -> w425
          shift-left: w404 -> [w768]
          tunnel: w403 -> [w767] mode=indexing
          n216 = call "ADCP_read_parameter.vi"("error in (no error)"=w769, "Parameter Name"=w767, "ADCP In"=w768) -> ("error out"=w771:errorcluster, "Parameter Value"=w770:string, "ADCP out"=w772:refnum<class "ADCP.lvclass">)  [unwired: 5 in, 1 out]
        }
        n217 = property class="LVClassControl (strict)"(reference=w426, "Value"=w425) -> (reference out=w424:refnum<vi>)  [unwired: 1 in, 1 out]
        n218 = Bundle By Name(cluster=w402, "ADCP"=w424) -> (w421:T1)
        n219 = for {
          tunnel: w419 -> [w432] mode=indexing
          shift-right: [w435] -> w422
          shift-left: w423 -> [w436]
          shift-right: [w433] -> w420
          shift-left: w421 -> [w434]
          i -> [w429]
          n220 = To Unsigned Word Integer(number=w429) -> (unsigned 16bit integer=w428:u16)
          n221 = Type Cast(type=MPU_Stick_Config_Parameters."IMU_ACCEL_FS" ("Enum"), x=w428) -> (*(type *) &x=w430:T10)
          n222 = case shown="\"MP_THRESHOLD_X_ACCEL_LOW\"" w430 {
            tunnel: w436 -> [w438 w443 w452 w462 w471 w481 w489 w497 w506 w515 w524 w532 w540 w548 w556 w564 w572 w580 w588 w596 w604 w612 w620 w628 w636 w644 w652 w660 w668 w676 w684 w693 w702 w711 w720 w729 w738 w747 w756 w765]
            tunnel: [w438 w442 w451 w461 w470 w480 w488 w496 w505 w514 w523 w531 w539 w547 w555 w563 w571 w579 w587 w595 w603 w611 w619 w627 w635 w643 w651 w659 w667 w675 w683 w692 w701 w710 w719 w728 w737 w746 w755 w764] -> w435
            tunnel: w434 -> [w437 w441 w450 w460 w469 w479 w487 w495 w504 w513 w522 w530 w538 w546 w554 w562 w570 w578 w586 w594 w602 w610 w618 w626 w634 w642 w650 w658 w666 w674 w682 w691 w700 w709 w718 w727 w736 w745 w754 w763]
            tunnel: [w437 w439 w448 w458 w467 w477 w485 w493 w502 w511 w520 w528 w536 w544 w552 w560 w568 w576 w584 w592 w600 w608 w616 w624 w632 w640 w648 w656 w664 w672 w680 w689 w698 w707 w716 w725 w734 w743 w752 w761] -> w433
            tunnel: w432 -> [_ w447 w456 w465 w474 w476 w484 w492 w500 w509 w518 w527 w535 w543 w551 w559 w567 w575 w583 w591 w599 w607 w615 w623 w631 w639 w647 w655 w663 w671 w679 w688 w697 w706 w715 w724 w733 w742 w751 w760]
            frame Default {
            }
            frame "IMU_ACCEL_FS" {
              n223 = Unbundle By Name(w441) -> ("IMU_configuration_references.IMU Accelerometer F.S. value"=w445:refnum<vi>)
              n224 = Search 1D Array(1D array=string[] ["IMU_ACCEL_FS_2G", "IMU_ACCEL_FS_4G", "IMU_ACCEL_FS_8G", "IMU_ACCEL_FS_16G"], element=w447) -> (index of element=w444:i32)  [unwired: 1 in]
              n225 = property class="Enum (strict)"(reference=w445, error in=w443, "Value"=w444) -> (reference out=w440:refnum<vi>, error out=w442:errorcluster)
              n226 = Bundle By Name(cluster=w441, "IMU_configuration_references.IMU Accelerometer F.S. value"=w440) -> (w439:T1)
            }
            frame "IMU_ACCEL_BW" {
              # "IMU_ACCEL_BW_460Hz:IMU_ACCEL_BW_184Hz:IMU_ACCEL_BW_92Hz:IMU_ACCEL_BW_41Hz:IMU_ACCEL_BW_20Hz:IMU_ACCEL_BW_10Hz:IMU_ACCEL_BW_5Hz"
              n227 = Unbundle By Name(w450) -> ("IMU_configuration_references.IMU Accelerometer bandwidth"=w454:refnum<vi>)
              n228 = Search 1D Array(1D array=string[] ["IMU_ACCEL_BW_460Hz", "IMU_ACCEL_BW_184Hz", "IMU_ACCEL_BW_92Hz", "IMU_ACCEL_BW_41Hz", "IMU_ACCEL_BW_20Hz", "IMU_ACCEL_BW_10Hz", "IMU_ACCEL_BW_5Hz"], element=w456) -> (index of element=w453:i32)  [unwired: 1 in]
              n229 = property class="Enum (strict)"(reference=w454, error in=w452, "Value"=w453) -> (reference out=w449:refnum<vi>, error out=w451:errorcluster)
              n230 = Bundle By Name(cluster=w450, "IMU_configuration_references.IMU Accelerometer bandwidth"=w449) -> (w448:T1)
            }
            frame "IMU_GYRO_FS" {
              # "IMU_GYRO_FS_250DPS:IMU_GYRO_FS_500DPS:IMU_GYRO_FS_1000DPS:IMU_GYRO_FS_2000DPS"
              n231 = Unbundle By Name(w460) -> ("IMU_configuration_references.IMU Gyroscope F.S. value"=w464:refnum<vi>)
              n232 = Search 1D Array(1D array=string[] ["IMU_GYRO_FS_250DPS", "IMU_GYRO_FS_500DPS", "IMU_GYRO_FS_1000DPS", "IMU_GYRO_FS_2000DPS"], element=w465) -> (index of element=w463:i32)  [unwired: 1 in]
              n233 = property class="Enum (strict)"(reference=w464, error in=w462, "Value"=w463) -> (reference out=w459:refnum<vi>, error out=w461:errorcluster)
              n234 = Bundle By Name(cluster=w460, "IMU_configuration_references.IMU Gyroscope F.S. value"=w459) -> (w458:T1)
            }
            frame "IMU_GYRO_BW" {
              # "IMU_GYRO_BW_NONE:IMU_GYRO_BW_184Hz:IMU_GYRO_BW_92Hz:IMU_GYRO_BW_41Hz:IMU_GYRO_BW_20Hz:IMU_GYRO_BW_10Hz:IMU_GYRO_BW_5Hz"
              n235 = Unbundle By Name(w469) -> ("IMU_configuration_references.IMU Gyroscope bandwidth"=w473:refnum<vi>)
              n236 = Search 1D Array(1D array=string[] ["IMU_GYRO_BW_NONE", "IMU_GYRO_BW_184Hz", "IMU_GYRO_BW_92Hz", "IMU_GYRO_BW_41Hz", "IMU_GYRO_BW_20Hz", "IMU_GYRO_BW_10Hz", "IMU_GYRO_BW_5Hz"], element=w474) -> (index of element=w472:i32)  [unwired: 1 in]
              n237 = property class="Enum (strict)"(reference=w473, error in=w471, "Value"=w472) -> (reference out=w468:refnum<vi>, error out=w470:errorcluster)
              n238 = Bundle By Name(cluster=w469, "IMU_configuration_references.IMU Gyroscope bandwidth"=w468) -> (w467:T1)
            }
            frame "IMU_CALIB_INTERVAL" {
              n239 = Unbundle By Name(w479) -> ("IMU_configuration_references.Calibration interval (ms)"=w482:refnum<vi>)
              n240 = Decimal String To Number(string=w476) -> (number=w475:i32)  [unwired: 2 in, 1 out]
              n241 = property class="DigNum (strict)"(reference=w482, error in=w481, "Value"=w475) -> (reference out=w478:refnum<vi>, error out=w480:errorcluster)
              n242 = Bundle By Name(cluster=w479, "IMU_configuration_references.Calibration interval (ms)"=w478) -> (w477:T1)
            }
            frame "IMU_CALIB_POINT_COUNT" {
              n243 = Unbundle By Name(w487) -> ("IMU_configuration_references.Calibration point count"=w490:refnum<vi>)
              n244 = Decimal String To Number(string=w484) -> (number=w483:i32)  [unwired: 2 in, 1 out]
              n245 = property class="DigNum (strict)"(reference=w490, error in=w489, "Value"=w483) -> (reference out=w486:refnum<vi>, error out=w488:errorcluster)
              n246 = Bundle By Name(cluster=w487, "IMU_configuration_references.Calibration point count"=w486) -> (w485:T1)
            }
            frame "IMU_SAMPLING_FREQ" {
              n247 = Unbundle By Name(w495) -> ("IMU_configuration_references.Sampling frequency (Hz)"=w498:refnum<vi>)
              n248 = Decimal String To Number(string=w492) -> (number=w491:i32)  [unwired: 2 in, 1 out]
              n249 = property class="DigNum (strict)"(reference=w498, error in=w497, "Value"=w491) -> (reference out=w494:refnum<vi>, error out=w496:errorcluster)
              n250 = Bundle By Name(cluster=w495, "IMU_configuration_references.Sampling frequency (Hz)"=w494) -> (w493:T1)
            }
            frame "LED1_CONFIG" {
              n251 = Unbundle By Name(w504) -> ("LED_Configuration_References.LED1 Configuration"=w507:refnum<vi>)
              n252 = Search 1D Array(1D array=string[] ["USER_CONTROLLED_DIG_OUTPUT", "X_ACCEL_PWM", "Y_ACCEL_PWM", "Z_ACCEL_PWM", "X_ACCEL_MD_OUTPUT", "Y_ACCEL_MD_OUTPUT", "Z_ACCEL_MD_OUTPUT", "X_GYRO_PWM", "Y_ACCEL_PWM", "Z_ACCEL_PWM", "X_GYRO_MD_OUTPUT", "Y_GYRO_MD_OUTPUT", "Z_GYRO_MD_OUTPUT", "ROLL_PWM", "PITCH_PWM", "YAW_PWM", "ROLL_MD_OUTPUT", "PITCH_MD_OUTPUT", "YAW_MD_OUTPUT", "USER_CONTROLLED_PWM_OUTPUT"] ("Array"), element=w500) -> (index of element=w499:i32)  [unwired: 1 in]
              n253 = property class="Enum (strict)"(reference=w507, error in=w506, "Value"=w499) -> (reference out=w503:refnum<vi>, error out=w505:errorcluster)
              n254 = Bundle By Name(cluster=w504, "LED_Configuration_References.LED1 Configuration"=w503) -> (w502:T1)
            }
            frame "LED2_CONFIG" {
              n255 = Unbundle By Name(w513) -> ("LED_Configuration_References.LED2 Configuration"=w516:refnum<vi>)
              n256 = Search 1D Array(1D array=string[] ["USER_CONTROLLED_DIG_OUTPUT", "X_ACCEL_PWM", "Y_ACCEL_PWM", "Z_ACCEL_PWM", "X_ACCEL_MD_OUTPUT", "Y_ACCEL_MD_OUTPUT", "Z_ACCEL_MD_OUTPUT", "X_GYRO_PWM", "Y_ACCEL_PWM", "Z_ACCEL_PWM", "X_GYRO_MD_OUTPUT", "Y_GYRO_MD_OUTPUT", "Z_GYRO_MD_OUTPUT", "ROLL_PWM", "PITCH_PWM", "YAW_PWM", "ROLL_MD_OUTPUT", "PITCH_MD_OUTPUT", "YAW_MD_OUTPUT", "USER_CONTROLLED_PWM_OUTPUT"] ("Array"), element=w509) -> (index of element=w508:i32)  [unwired: 1 in]
              n257 = property class="Enum (strict)"(reference=w516, error in=w515, "Value"=w508) -> (reference out=w512:refnum<vi>, error out=w514:errorcluster)
              n258 = Bundle By Name(cluster=w513, "LED_Configuration_References.LED2 Configuration"=w512) -> (w511:T1)
            }
            frame "LED3_CONFIG" {
              n259 = Unbundle By Name(w522) -> ("LED_Configuration_References.LED3 Configuration"=w525:refnum<vi>)
              n260 = Search 1D Array(1D array=string[] ["USER_CONTROLLED_DIG_OUTPUT", "X_ACCEL_PWM", "Y_ACCEL_PWM", "Z_ACCEL_PWM", "X_ACCEL_MD_OUTPUT", "Y_ACCEL_MD_OUTPUT", "Z_ACCEL_MD_OUTPUT", "X_GYRO_PWM", "Y_ACCEL_PWM", "Z_ACCEL_PWM", "X_GYRO_MD_OUTPUT", "Y_GYRO_MD_OUTPUT", "Z_GYRO_MD_OUTPUT", "ROLL_PWM", "PITCH_PWM", "YAW_PWM", "ROLL_MD_OUTPUT", "PITCH_MD_OUTPUT", "YAW_MD_OUTPUT", "USER_CONTROLLED_PWM_OUTPUT"] ("Array"), element=w518) -> (index of element=w517:i32)  [unwired: 1 in]
              n261 = property class="Enum (strict)"(reference=w525, error in=w524, "Value"=w517) -> (reference out=w521:refnum<vi>, error out=w523:errorcluster)
              n262 = Bundle By Name(cluster=w522, "LED_Configuration_References.LED3 Configuration"=w521) -> (w520:T1)
            }
            frame "MP_ROLL_FILTER_CONSTANT" {
              n263 = Unbundle By Name(w530) -> ("MP_Comp_Filter_Constants_References.Roll filter constant"=w533:refnum<vi>)
              n264 = Fract/Exp String To Number(string=w527) -> (number=w526:dbl)  [unwired: 3 in, 1 out]
              n265 = property class="DigNum (strict)"(reference=w533, error in=w532, "Value"=w526) -> (reference out=w529:refnum<vi>, error out=w531:errorcluster)
              n266 = Bundle By Name(cluster=w530, "MP_Comp_Filter_Constants_References.Roll filter constant"=w529) -> (w528:T1)
            }
            frame "MP_PITCH_FILTER_CONSTANT" {
              n267 = Unbundle By Name(w538) -> ("MP_Comp_Filter_Constants_References.Pitch filter constant"=w541:refnum<vi>)
              n268 = Fract/Exp String To Number(string=w535) -> (number=w534:dbl)  [unwired: 3 in, 1 out]
              n269 = property class="DigNum (strict)"(reference=w541, error in=w540, "Value"=w534) -> (reference out=w537:refnum<vi>, error out=w539:errorcluster)
              n270 = Bundle By Name(cluster=w538, "MP_Comp_Filter_Constants_References.Pitch filter constant"=w537) -> (w536:T1)
            }
            frame "MP_THRESHOLD_X_ACCEL_LOW" {
              n271 = Unbundle By Name(w546) -> ("MD_Threshold_References.X accel. threshold (L)"=w549:refnum<vi>)
              n272 = Fract/Exp String To Number(string=w543) -> (number=w542:dbl)  [unwired: 3 in, 1 out]
              n273 = property class="DigNum (strict)"(reference=w549, error in=w548, "Value"=w542) -> (reference out=w545:refnum<vi>, error out=w547:errorcluster)
              n274 = Bundle By Name(cluster=w546, "MD_Threshold_References.X accel. threshold (L)"=w545) -> (w544:T1)
            }
            frame "MP_THRESHOLD_X_ACCEL_HIGH" {
              n275 = Unbundle By Name(w554) -> ("MD_Threshold_References.X accel. threshold (U)"=w557:refnum<vi>)
              n276 = Fract/Exp String To Number(string=w551) -> (number=w550:dbl)  [unwired: 3 in, 1 out]
              n277 = property class="DigNum (strict)"(reference=w557, error in=w556, "Value"=w550) -> (reference out=w553:refnum<vi>, error out=w555:errorcluster)
              n278 = Bundle By Name(cluster=w554, "MD_Threshold_References.X accel. threshold (U)"=w553) -> (w552:T1)
            }
            frame "MP_THRESHOLD_Y_ACCEL_LOW" {
              n279 = Unbundle By Name(w562) -> ("MD_Threshold_References.Y accel. threshold (L)"=w565:refnum<vi>)
              n280 = Fract/Exp String To Number(string=w559) -> (number=w558:dbl)  [unwired: 3 in, 1 out]
              n281 = property class="DigNum (strict)"(reference=w565, error in=w564, "Value"=w558) -> (reference out=w561:refnum<vi>, error out=w563:errorcluster)
              n282 = Bundle By Name(cluster=w562, "MD_Threshold_References.Y accel. threshold (L)"=w561) -> (w560:T1)
            }
            frame "MP_THRESHOLD_Y_ACCEL_HIGH" {
              n283 = Unbundle By Name(w570) -> ("MD_Threshold_References.Y accel. threshold (U)"=w573:refnum<vi>)
              n284 = Fract/Exp String To Number(string=w567) -> (number=w566:dbl)  [unwired: 3 in, 1 out]
              n285 = property class="DigNum (strict)"(reference=w573, error in=w572, "Value"=w566) -> (reference out=w569:refnum<vi>, error out=w571:errorcluster)
              n286 = Bundle By Name(cluster=w570, "MD_Threshold_References.Y accel. threshold (U)"=w569) -> (w568:T1)
            }
            frame "MP_THRESHOLD_Z_ACCEL_LOW" {
              n287 = Unbundle By Name(w578) -> ("MD_Threshold_References.Z accel. threshold (L)"=w581:refnum<vi>)
              n288 = Fract/Exp String To Number(string=w575) -> (number=w574:dbl)  [unwired: 3 in, 1 out]
              n289 = property class="DigNum (strict)"(reference=w581, error in=w580, "Value"=w574) -> (reference out=w577:refnum<vi>, error out=w579:errorcluster)
              n290 = Bundle By Name(cluster=w578, "MD_Threshold_References.Z accel. threshold (L)"=w577) -> (w576:T1)
            }
            frame "MP_THRESHOLD_Z_ACCEL_HIGH" {
              n291 = Unbundle By Name(w586) -> ("MD_Threshold_References.Z accel. threshold (U)"=w589:refnum<vi>)
              n292 = Fract/Exp String To Number(string=w583) -> (number=w582:dbl)  [unwired: 3 in, 1 out]
              n293 = property class="DigNum (strict)"(reference=w589, error in=w588, "Value"=w582) -> (reference out=w585:refnum<vi>, error out=w587:errorcluster)
              n294 = Bundle By Name(cluster=w586, "MD_Threshold_References.Z accel. threshold (U)"=w585) -> (w584:T1)
            }
            frame "MP_THRESHOLD_X_GYRO_LOW" {
              n295 = Unbundle By Name(w594) -> ("MD_Threshold_References.X gyro. threshold (L)"=w597:refnum<vi>)
              n296 = Fract/Exp String To Number(string=w591) -> (number=w590:dbl)  [unwired: 3 in, 1 out]
              n297 = property class="DigNum (strict)"(reference=w597, error in=w596, "Value"=w590) -> (reference out=w593:refnum<vi>, error out=w595:errorcluster)
              n298 = Bundle By Name(cluster=w594, "MD_Threshold_References.X gyro. threshold (L)"=w593) -> (w592:T1)
            }
            frame "MP_THRESHOLD_X_GYRO_HIGH" {
              n299 = Unbundle By Name(w602) -> ("MD_Threshold_References.X gyro. threshold (U)"=w605:refnum<vi>)
              n300 = Fract/Exp String To Number(string=w599) -> (number=w598:dbl)  [unwired: 3 in, 1 out]
              n301 = property class="DigNum (strict)"(reference=w605, error in=w604, "Value"=w598) -> (reference out=w601:refnum<vi>, error out=w603:errorcluster)
              n302 = Bundle By Name(cluster=w602, "MD_Threshold_References.X gyro. threshold (U)"=w601) -> (w600:T1)
            }
            frame "MP_THRESHOLD_Y_GYRO_LOW" {
              n303 = Unbundle By Name(w610) -> ("MD_Threshold_References.Y gyro. threshold (L)"=w613:refnum<vi>)
              n304 = Fract/Exp String To Number(string=w607) -> (number=w606:dbl)  [unwired: 3 in, 1 out]
              n305 = property class="DigNum (strict)"(reference=w613, error in=w612, "Value"=w606) -> (reference out=w609:refnum<vi>, error out=w611:errorcluster)
              n306 = Bundle By Name(cluster=w610, "MD_Threshold_References.Y gyro. threshold (L)"=w609) -> (w608:T1)
            }
            frame "MP_THRESHOLD_Y_GYRO_HIGH" {
              n307 = Unbundle By Name(w618) -> ("MD_Threshold_References.Y gyro. threshold (U)"=w621:refnum<vi>)
              n308 = Fract/Exp String To Number(string=w615) -> (number=w614:dbl)  [unwired: 3 in, 1 out]
              n309 = property class="DigNum (strict)"(reference=w621, error in=w620, "Value"=w614) -> (reference out=w617:refnum<vi>, error out=w619:errorcluster)
              n310 = Bundle By Name(cluster=w618, "MD_Threshold_References.Y gyro. threshold (U)"=w617) -> (w616:T1)
            }
            frame "MP_THRESHOLD_Z_GYRO_LOW" {
              n311 = Unbundle By Name(w626) -> ("MD_Threshold_References.Z gyro. threshold (L)"=w629:refnum<vi>)
              n312 = Fract/Exp String To Number(string=w623) -> (number=w622:dbl)  [unwired: 3 in, 1 out]
              n313 = property class="DigNum (strict)"(reference=w629, error in=w628, "Value"=w622) -> (reference out=w625:refnum<vi>, error out=w627:errorcluster)
              n314 = Bundle By Name(cluster=w626, "MD_Threshold_References.Z gyro. threshold (L)"=w625) -> (w624:T1)
            }
            frame "MP_THRESHOLD_Z_GYRO_HIGH" {
              n315 = Unbundle By Name(w634) -> ("MD_Threshold_References.Z gyro. threshold (U)"=w637:refnum<vi>)
              n316 = Fract/Exp String To Number(string=w631) -> (number=w630:dbl)  [unwired: 3 in, 1 out]
              n317 = property class="DigNum (strict)"(reference=w637, error in=w636, "Value"=w630) -> (reference out=w633:refnum<vi>, error out=w635:errorcluster)
              n318 = Bundle By Name(cluster=w634, "MD_Threshold_References.Z gyro. threshold (U)"=w633) -> (w632:T1)
            }
            frame "MP_THRESHOLD_ROLL_LOW" {
              n319 = Unbundle By Name(w642) -> ("MD_Threshold_References.Roll threshold (L)"=w645:refnum<vi>)
              n320 = Fract/Exp String To Number(string=w639) -> (number=w638:dbl)  [unwired: 3 in, 1 out]
              n321 = property class="DigNum (strict)"(reference=w645, error in=w644, "Value"=w638) -> (reference out=w641:refnum<vi>, error out=w643:errorcluster)
              n322 = Bundle By Name(cluster=w642, "MD_Threshold_References.Roll threshold (L)"=w641) -> (w640:T1)
            }
            frame "MP_THRESHOLD_ROLL_HIGH" {
              n323 = Unbundle By Name(w650) -> ("MD_Threshold_References.Roll threshold (U)"=w653:refnum<vi>)
              n324 = Fract/Exp String To Number(string=w647) -> (number=w646:dbl)  [unwired: 3 in, 1 out]
              n325 = property class="DigNum (strict)"(reference=w653, error in=w652, "Value"=w646) -> (reference out=w649:refnum<vi>, error out=w651:errorcluster)
              n326 = Bundle By Name(cluster=w650, "MD_Threshold_References.Roll threshold (U)"=w649) -> (w648:T1)
            }
            frame "MP_THRESHOLD_PITCH_LOW" {
              n327 = Unbundle By Name(w658) -> ("MD_Threshold_References.Pitch. threshold (L)"=w661:refnum<vi>)
              n328 = Fract/Exp String To Number(string=w655) -> (number=w654:dbl)  [unwired: 3 in, 1 out]
              n329 = property class="DigNum (strict)"(reference=w661, error in=w660, "Value"=w654) -> (reference out=w657:refnum<vi>, error out=w659:errorcluster)
              n330 = Bundle By Name(cluster=w658, "MD_Threshold_References.Pitch. threshold (L)"=w657) -> (w656:T1)
            }
            frame "MP_THRESHOLD_PITCH_HIGH" {
              n331 = Unbundle By Name(w666) -> ("MD_Threshold_References.Pitch threshold (U)"=w669:refnum<vi>)
              n332 = Fract/Exp String To Number(string=w663) -> (number=w662:dbl)  [unwired: 3 in, 1 out]
              n333 = property class="DigNum (strict)"(reference=w669, error in=w668, "Value"=w662) -> (reference out=w665:refnum<vi>, error out=w667:errorcluster)
              n334 = Bundle By Name(cluster=w666, "MD_Threshold_References.Pitch threshold (U)"=w665) -> (w664:T1)
            }
            frame "MP_THRESHOLD_YAW_LOW" {
              n335 = Unbundle By Name(w674) -> ("MD_Threshold_References.Yaw threshold (L)"=w677:refnum<vi>)
              n336 = Fract/Exp String To Number(string=w671) -> (number=w670:dbl)  [unwired: 3 in, 1 out]
              n337 = property class="DigNum (strict)"(reference=w677, error in=w676, "Value"=w670) -> (reference out=w673:refnum<vi>, error out=w675:errorcluster)
              n338 = Bundle By Name(cluster=w674, "MD_Threshold_References.Yaw threshold (L)"=w673) -> (w672:T1)
            }
            frame "MP_THRESHOLD_YAW_HIGH" {
              n339 = Unbundle By Name(w682) -> ("MD_Threshold_References.Yaw threshold (U)"=w685:refnum<vi>)
              n340 = Fract/Exp String To Number(string=w679) -> (number=w678:dbl)  [unwired: 3 in, 1 out]
              n341 = property class="DigNum (strict)"(reference=w685, error in=w684, "Value"=w678) -> (reference out=w681:refnum<vi>, error out=w683:errorcluster)
              n342 = Bundle By Name(cluster=w682, "MD_Threshold_References.Yaw threshold (U)"=w681) -> (w680:T1)
            }
            frame "MP_DETECTION_TYPE_X_ACCEL" {
              n343 = Unbundle By Name(w691) -> ("MD_Type_References.X accel threshold type"=w694:refnum<vi>)
              n344 = Search 1D Array(1D array=string[] ["ABS_LESSER_THAN", "ABS_GREATER_THAN", "LESSER_THAN", "GREATER_THAN", "WINDOWED_MODE_WITHIN_BOUNDS", "WINDOWED_MODE_OUTSIDE_BOUNDS"] ("Array"), element=w688) -> (index of element=w687:i32)  [unwired: 1 in]
              n345 = property class="Enum (strict)"(reference=w694, error in=w693, "Value"=w687) -> (reference out=w690:refnum<vi>, error out=w692:errorcluster)
              n346 = Bundle By Name(cluster=w691, "MD_Type_References.X accel threshold type"=w690) -> (w689:T1)
            }
            frame "MP_DETECTION_TYPE_Y_ACCEL" {
              n347 = Unbundle By Name(w700) -> ("MD_Type_References.Y accel threshold type"=w703:refnum<vi>)
              n348 = Search 1D Array(1D array=string[] ["ABS_LESSER_THAN", "ABS_GREATER_THAN", "LESSER_THAN", "GREATER_THAN", "WINDOWED_MODE_WITHIN_BOUNDS", "WINDOWED_MODE_OUTSIDE_BOUNDS"] ("Array"), element=w697) -> (index of element=w696:i32)  [unwired: 1 in]
              n349 = property class="Enum (strict)"(reference=w703, error in=w702, "Value"=w696) -> (reference out=w699:refnum<vi>, error out=w701:errorcluster)
              n350 = Bundle By Name(cluster=w700, "MD_Type_References.Y accel threshold type"=w699) -> (w698:T1)
            }
            frame "MP_DETECTION_TYPE_Z_ACCEL" {
              n351 = Unbundle By Name(w709) -> ("MD_Type_References.Z accel threshold type"=w712:refnum<vi>)
              n352 = Search 1D Array(1D array=string[] ["ABS_LESSER_THAN", "ABS_GREATER_THAN", "LESSER_THAN", "GREATER_THAN", "WINDOWED_MODE_WITHIN_BOUNDS", "WINDOWED_MODE_OUTSIDE_BOUNDS"] ("Array"), element=w706) -> (index of element=w705:i32)  [unwired: 1 in]
              n353 = property class="Enum (strict)"(reference=w712, error in=w711, "Value"=w705) -> (reference out=w708:refnum<vi>, error out=w710:errorcluster)
              n354 = Bundle By Name(cluster=w709, "MD_Type_References.Z accel threshold type"=w708) -> (w707:T1)
            }
            frame "MP_DETECTION_TYPE_X_GYRO" {
              n355 = Unbundle By Name(w718) -> ("MD_Type_References.X gyro threshold type"=w721:refnum<vi>)
              n356 = Search 1D Array(1D array=string[] ["ABS_LESSER_THAN", "ABS_GREATER_THAN", "LESSER_THAN", "GREATER_THAN", "WINDOWED_MODE_WITHIN_BOUNDS", "WINDOWED_MODE_OUTSIDE_BOUNDS"] ("Array"), element=w715) -> (index of element=w714:i32)  [unwired: 1 in]
              n357 = property class="Enum (strict)"(reference=w721, error in=w720, "Value"=w714) -> (reference out=w717:refnum<vi>, error out=w719:errorcluster)
              n358 = Bundle By Name(cluster=w718, "MD_Type_References.X gyro threshold type"=w717) -> (w716:T1)
            }
            frame "MP_DETECTION_TYPE_Y_GYRO" {
              n359 = Unbundle By Name(w727) -> ("MD_Type_References.Y gyro threshold type"=w730:refnum<vi>)
              n360 = Search 1D Array(1D array=string[] ["ABS_LESSER_THAN", "ABS_GREATER_THAN", "LESSER_THAN", "GREATER_THAN", "WINDOWED_MODE_WITHIN_BOUNDS", "WINDOWED_MODE_OUTSIDE_BOUNDS"] ("Array"), element=w724) -> (index of element=w723:i32)  [unwired: 1 in]
              n361 = property class="Enum (strict)"(reference=w730, error in=w729, "Value"=w723) -> (reference out=w726:refnum<vi>, error out=w728:errorcluster)
              n362 = Bundle By Name(cluster=w727, "MD_Type_References.Y gyro threshold type"=w726) -> (w725:T1)
            }
            frame "MP_DETECTION_TYPE_Z_GYRO" {
              n363 = Unbundle By Name(w736) -> ("MD_Type_References.Z gyro threshold type"=w739:refnum<vi>)
              n364 = Search 1D Array(1D array=string[] ["ABS_LESSER_THAN", "ABS_GREATER_THAN", "LESSER_THAN", "GREATER_THAN", "WINDOWED_MODE_WITHIN_BOUNDS", "WINDOWED_MODE_OUTSIDE_BOUNDS"] ("Array"), element=w733) -> (index of element=w732:i32)  [unwired: 1 in]
              n365 = property class="Enum (strict)"(reference=w739, error in=w738, "Value"=w732) -> (reference out=w735:refnum<vi>, error out=w737:errorcluster)
              n366 = Bundle By Name(cluster=w736, "MD_Type_References.Z gyro threshold type"=w735) -> (w734:T1)
            }
            frame "MP_DETECTION_TYPE_ROLL" {
              n367 = Unbundle By Name(w745) -> ("MD_Type_References.Roll threshold type"=w748:refnum<vi>)
              n368 = Search 1D Array(1D array=string[] ["ABS_LESSER_THAN", "ABS_GREATER_THAN", "LESSER_THAN", "GREATER_THAN", "WINDOWED_MODE_WITHIN_BOUNDS", "WINDOWED_MODE_OUTSIDE_BOUNDS"] ("Array"), element=w742) -> (index of element=w741:i32)  [unwired: 1 in]
              n369 = property class="Enum (strict)"(reference=w748, error in=w747, "Value"=w741) -> (reference out=w744:refnum<vi>, error out=w746:errorcluster)
              n370 = Bundle By Name(cluster=w745, "MD_Type_References.Roll threshold type"=w744) -> (w743:T1)
            }
            frame "MP_DETECTION_TYPE_PITCH" {
              n371 = Unbundle By Name(w754) -> ("MD_Type_References.Pitch threshold type"=w757:refnum<vi>)
              n372 = Search 1D Array(1D array=string[] ["ABS_LESSER_THAN", "ABS_GREATER_THAN", "LESSER_THAN", "GREATER_THAN", "WINDOWED_MODE_WITHIN_BOUNDS", "WINDOWED_MODE_OUTSIDE_BOUNDS"] ("Array"), element=w751) -> (index of element=w750:i32)  [unwired: 1 in]
              n373 = property class="Enum (strict)"(reference=w757, error in=w756, "Value"=w750) -> (reference out=w753:refnum<vi>, error out=w755:errorcluster)
              n374 = Bundle By Name(cluster=w754, "MD_Type_References.Pitch threshold type"=w753) -> (w752:T1)
            }
            frame "MP_DETECTION_TYPE_YAW" {
              n375 = Unbundle By Name(w763) -> ("MD_Type_References.Yaw threshold type"=w766:refnum<vi>)
              n376 = Search 1D Array(1D array=string[] ["ABS_LESSER_THAN", "ABS_GREATER_THAN", "LESSER_THAN", "GREATER_THAN", "WINDOWED_MODE_WITHIN_BOUNDS", "WINDOWED_MODE_OUTSIDE_BOUNDS"] ("Array"), element=w760) -> (index of element=w759:i32)  [unwired: 1 in]
              n377 = property class="Enum (strict)"(reference=w766, error in=w765, "Value"=w759) -> (reference out=w762:refnum<vi>, error out=w764:errorcluster)
              n378 = Bundle By Name(cluster=w763, "MD_Type_References.Yaw threshold type"=w762) -> (w761:T1)
            }
          }
        }
      }
      frame "Write" {
        n379 = case shown="\"IMU_ACCEL_FS\"" w837 {
          tunnel: w838 -> [w841 w848 w855 w862 w869 w875 w881 w887 w894 w901 w908 w914 w920 w926 w932 w938 w944 w950 w956 w962 w968 w974 w980 w986 w992 w998 w1004 w1010 w1016 w1022 w1028 w1035 w1042 w1049 w1056 w1063 w1070 w1077 w1084 w1091]
          tunnel: [w841 w848 w855 w862 w869 w875 w881 w887 w894 w901 w908 w914 w920 w926 w932 w938 w944 w950 w956 w962 w968 w974 w980 w986 w992 w998 w1004 w1010 w1016 w1022 w1028 w1035 w1042 w1049 w1056 w1063 w1070 w1077 w1084 w1091] -> w833
          tunnel: w836 -> [w840 w847 w854 w861 w868 w874 w880 w886 w893 w900 w907 w913 w919 w925 w931 w937 w943 w949 w955 w961 w967 w973 w979 w985 w991 w997 w1003 w1009 w1015 w1021 w1027 w1034 w1041 w1048 w1055 w1062 w1069 w1076 w1083 w1090]
          tunnel: [w840 w845 w852 w859 w866 w872 w878 w884 w891 w898 w905 w911 w917 w923 w929 w935 w941 w947 w953 w959 w965 w971 w977 w983 w989 w995 w1001 w1007 w1013 w1019 w1025 w1032 w1039 w1046 w1053 w1060 w1067 w1074 w1081 w1088] -> w830
          tunnel: ["" w842 w849 w856 w864 w870 w876 w882 w888 w895 w902 w909 w915 w921 w927 w933 w939 w945 w951 w957 w963 w969 w975 w981 w987 w993 w999 w1005 w1011 w1017 w1023 w1029 w1036 w1043 w1050 w1057 w1064 w1071 w1078 w1085] -> w826
          frame Default {
          }
          frame "IMU_ACCEL_FS" {
            n380 = Unbundle By Name(w848) -> ("IMU_configuration_references.IMU Accelerometer F.S. value"=w846:refnum<vi>)
            n381 = property class="Enum (strict)"(reference=w846, error in=w847) -> (error out=w845:errorcluster, "Value"=w843:T12)  [unwired: 1 out]
            n382 = Index Array(array=string[] ["IMU_ACCEL_FS_2G", "IMU_ACCEL_FS_4G", "IMU_ACCEL_FS_8G", "IMU_ACCEL_FS_16G"], index=w843) -> (element=w842:string)
          }
          frame "IMU_ACCEL_BW" {
            n383 = Unbundle By Name(w855) -> ("IMU_configuration_references.IMU Accelerometer bandwidth"=w853:refnum<vi>)
            n384 = property class="Enum (strict)"(reference=w853, error in=w854) -> (error out=w852:errorcluster, "Value"=w851:T13)  [unwired: 1 out]
            n385 = Index Array(array=string[] ["IMU_ACCEL_BW_460Hz", "IMU_ACCEL_BW_184Hz", "IMU_ACCEL_BW_92Hz", "IMU_ACCEL_BW_41Hz", "IMU_ACCEL_BW_20Hz", "IMU_ACCEL_BW_10Hz", "IMU_ACCEL_BW_5Hz"], index=w851) -> (element=w849:string)
          }
          frame "IMU_GYRO_FS" {
            n386 = Unbundle By Name(w862) -> ("IMU_configuration_references.IMU Gyroscope F.S. value"=w860:refnum<vi>)
            n387 = property class="Enum (strict)"(reference=w860, error in=w861) -> (error out=w859:errorcluster, "Value"=w858:T14)  [unwired: 1 out]
            n388 = Index Array(array=string[] ["IMU_GYRO_FS_250DPS", "IMU_GYRO_FS_500DPS", "IMU_GYRO_FS_1000DPS", "IMU_GYRO_FS_2000DPS"] ("1D array"), index=w858) -> (element=w856:string)
          }
          frame "IMU_GYRO_BW" {
            n389 = Unbundle By Name(w869) -> ("IMU_configuration_references.IMU Gyroscope bandwidth"=w867:refnum<vi>)
            n390 = property class="Enum (strict)"(reference=w867, error in=w868) -> (error out=w866:errorcluster, "Value"=w865:T15)  [unwired: 1 out]
            n391 = Index Array(array=string[] ["IMU_GYRO_BW_NONE", "IMU_GYRO_BW_184Hz", "IMU_GYRO_BW_92Hz", "IMU_GYRO_BW_41Hz", "IMU_GYRO_BW_20Hz", "IMU_GYRO_BW_10Hz", "IMU_GYRO_BW_5Hz"] ("1D array"), index=w865) -> (element=w864:string)
          }
          frame "IMU_CALIB_INTERVAL" {
            n392 = Unbundle By Name(w875) -> ("IMU_configuration_references.Calibration interval (ms)"=w873:refnum<vi>)
            n393 = property class="DigNum (strict)"(reference=w873, error in=w874) -> (error out=w872:errorcluster, "Value"=w871:u16)  [unwired: 1 out]
            n394 = Number To Decimal String(number=w871) -> (decimal integer string=w870:string)  [unwired: 1 in]
          }
          frame "IMU_CALIB_POINT_COUNT" {
            n395 = Unbundle By Name(w881) -> ("IMU_configuration_references.Calibration point count"=w879:refnum<vi>)
            n396 = property class="DigNum (strict)"(reference=w879, error in=w880) -> (error out=w878:errorcluster, "Value"=w877:u16)  [unwired: 1 out]
            n397 = Number To Decimal String(number=w877) -> (decimal integer string=w876:string)  [unwired: 1 in]
          }
          frame "IMU_SAMPLING_FREQ" {
            n398 = Unbundle By Name(w887) -> ("IMU_configuration_references.Sampling frequency (Hz)"=w885:refnum<vi>)
            n399 = property class="DigNum (strict)"(reference=w885, error in=w886) -> (error out=w884:errorcluster, "Value"=w883:u16)  [unwired: 1 out]
            n400 = Number To Decimal String(number=w883) -> (decimal integer string=w882:string)  [unwired: 1 in]
          }
          frame "LED1_CONFIG" {
            n401 = Unbundle By Name(w894) -> ("LED_Configuration_References.LED1 Configuration"=w892:refnum<vi>)
            n402 = property class="Enum (strict)"(reference=w892, error in=w893) -> (error out=w891:errorcluster, "Value"=w889:T16)  [unwired: 1 out]
            n403 = Index Array(array=string[] ["USER_CONTROLLED_DIG_OUTPUT", "X_ACCEL_PWM", "Y_ACCEL_PWM", "Z_ACCEL_PWM", "X_ACCEL_MD_OUTPUT", "Y_ACCEL_MD_OUTPUT", "Z_ACCEL_MD_OUTPUT", "X_GYRO_PWM", "Y_ACCEL_PWM", "Z_ACCEL_PWM", "X_GYRO_MD_OUTPUT", "Y_GYRO_MD_OUTPUT", "Z_GYRO_MD_OUTPUT", "ROLL_PWM", "PITCH_PWM", "YAW_PWM", "ROLL_MD_OUTPUT", "PITCH_MD_OUTPUT", "YAW_MD_OUTPUT", "USER_CONTROLLED_PWM_OUTPUT"] ("Array"), index=w889) -> (element=w888:string)
          }
          frame "LED2_CONFIG" {
            n404 = Unbundle By Name(w901) -> ("LED_Configuration_References.LED2 Configuration"=w899:refnum<vi>)
            n405 = property class="Enum (strict)"(reference=w899, error in=w900) -> (error out=w898:errorcluster, "Value"=w896:T16)  [unwired: 1 out]
            n406 = Index Array(array=string[] ["USER_CONTROLLED_DIG_OUTPUT", "X_ACCEL_PWM", "Y_ACCEL_PWM", "Z_ACCEL_PWM", "X_ACCEL_MD_OUTPUT", "Y_ACCEL_MD_OUTPUT", "Z_ACCEL_MD_OUTPUT", "X_GYRO_PWM", "Y_ACCEL_PWM", "Z_ACCEL_PWM", "X_GYRO_MD_OUTPUT", "Y_GYRO_MD_OUTPUT", "Z_GYRO_MD_OUTPUT", "ROLL_PWM", "PITCH_PWM", "YAW_PWM", "ROLL_MD_OUTPUT", "PITCH_MD_OUTPUT", "YAW_MD_OUTPUT", "USER_CONTROLLED_PWM_OUTPUT"] ("Array"), index=w896) -> (element=w895:string)
          }
          frame "LED3_CONFIG" {
            n407 = Unbundle By Name(w908) -> ("LED_Configuration_References.LED3 Configuration"=w906:refnum<vi>)
            n408 = property class="Enum (strict)"(reference=w906, error in=w907) -> (error out=w905:errorcluster, "Value"=w903:T16)  [unwired: 1 out]
            n409 = Index Array(array=string[] ["USER_CONTROLLED_DIG_OUTPUT", "X_ACCEL_PWM", "Y_ACCEL_PWM", "Z_ACCEL_PWM", "X_ACCEL_MD_OUTPUT", "Y_ACCEL_MD_OUTPUT", "Z_ACCEL_MD_OUTPUT", "X_GYRO_PWM", "Y_ACCEL_PWM", "Z_ACCEL_PWM", "X_GYRO_MD_OUTPUT", "Y_GYRO_MD_OUTPUT", "Z_GYRO_MD_OUTPUT", "ROLL_PWM", "PITCH_PWM", "YAW_PWM", "ROLL_MD_OUTPUT", "PITCH_MD_OUTPUT", "YAW_MD_OUTPUT", "USER_CONTROLLED_PWM_OUTPUT"] ("Array"), index=w903) -> (element=w902:string)
          }
          frame "MP_ROLL_FILTER_CONSTANT" {
            n410 = Unbundle By Name(w914) -> ("MP_Comp_Filter_Constants_References.Roll filter constant"=w912:refnum<vi>)
            n411 = property class="DigNum (strict)"(reference=w912, error in=w913) -> (error out=w911:errorcluster, "Value"=w910:dbl)  [unwired: 1 out]
            n412 = Number To Fractional String(number=w910) -> (F-format string=w909:string)  [unwired: 3 in]
          }
          frame "MP_PITCH_FILTER_CONSTANT" {
            n413 = Unbundle By Name(w920) -> ("MP_Comp_Filter_Constants_References.Pitch filter constant"=w918:refnum<vi>)
            n414 = property class="DigNum (strict)"(reference=w918, error in=w919) -> (error out=w917:errorcluster, "Value"=w916:dbl)  [unwired: 1 out]
            n415 = Number To Fractional String(number=w916) -> (F-format string=w915:string)  [unwired: 3 in]
          }
          frame "MP_THRESHOLD_X_ACCEL_LOW" {
            n416 = Unbundle By Name(w926) -> ("MD_Threshold_References.X accel. threshold (L)"=w924:refnum<vi>)
            n417 = property class="DigNum (strict)"(reference=w924, error in=w925) -> (error out=w923:errorcluster, "Value"=w922:dbl)  [unwired: 1 out]
            n418 = Number To Fractional String(number=w922) -> (F-format string=w921:string)  [unwired: 3 in]
          }
          frame "MP_THRESHOLD_X_ACCEL_HIGH" {
            n419 = Unbundle By Name(w932) -> ("MD_Threshold_References.X accel. threshold (U)"=w930:refnum<vi>)
            n420 = property class="DigNum (strict)"(reference=w930, error in=w931) -> (error out=w929:errorcluster, "Value"=w928:dbl)  [unwired: 1 out]
            n421 = Number To Fractional String(number=w928) -> (F-format string=w927:string)  [unwired: 3 in]
          }
          frame "MP_THRESHOLD_Y_ACCEL_LOW" {
            n422 = Unbundle By Name(w938) -> ("MD_Threshold_References.Y accel. threshold (L)"=w936:refnum<vi>)
            n423 = property class="DigNum (strict)"(reference=w936, error in=w937) -> (error out=w935:errorcluster, "Value"=w934:dbl)  [unwired: 1 out]
            n424 = Number To Fractional String(number=w934) -> (F-format string=w933:string)  [unwired: 3 in]
          }
          frame "MP_THRESHOLD_Y_ACCEL_HIGH" {
            n425 = Unbundle By Name(w944) -> ("MD_Threshold_References.Y accel. threshold (U)"=w942:refnum<vi>)
            n426 = property class="DigNum (strict)"(reference=w942, error in=w943) -> (error out=w941:errorcluster, "Value"=w940:dbl)  [unwired: 1 out]
            n427 = Number To Fractional String(number=w940) -> (F-format string=w939:string)  [unwired: 3 in]
          }
          frame "MP_THRESHOLD_Z_ACCEL_LOW" {
            n428 = Unbundle By Name(w950) -> ("MD_Threshold_References.Z accel. threshold (L)"=w948:refnum<vi>)
            n429 = property class="DigNum (strict)"(reference=w948, error in=w949) -> (error out=w947:errorcluster, "Value"=w946:dbl)  [unwired: 1 out]
            n430 = Number To Fractional String(number=w946) -> (F-format string=w945:string)  [unwired: 3 in]
          }
          frame "MP_THRESHOLD_Z_ACCEL_HIGH" {
            n431 = Unbundle By Name(w956) -> ("MD_Threshold_References.Z accel. threshold (U)"=w954:refnum<vi>)
            n432 = property class="DigNum (strict)"(reference=w954, error in=w955) -> (error out=w953:errorcluster, "Value"=w952:dbl)  [unwired: 1 out]
            n433 = Number To Fractional String(number=w952) -> (F-format string=w951:string)  [unwired: 3 in]
          }
          frame "MP_THRESHOLD_X_GYRO_LOW" {
            n434 = Unbundle By Name(w962) -> ("MD_Threshold_References.X gyro. threshold (L)"=w960:refnum<vi>)
            n435 = property class="DigNum (strict)"(reference=w960, error in=w961) -> (error out=w959:errorcluster, "Value"=w958:dbl)  [unwired: 1 out]
            n436 = Number To Fractional String(number=w958) -> (F-format string=w957:string)  [unwired: 3 in]
          }
          frame "MP_THRESHOLD_X_GYRO_HIGH" {
            n437 = Unbundle By Name(w968) -> ("MD_Threshold_References.X gyro. threshold (U)"=w966:refnum<vi>)
            n438 = property class="DigNum (strict)"(reference=w966, error in=w967) -> (error out=w965:errorcluster, "Value"=w964:dbl)  [unwired: 1 out]
            n439 = Number To Fractional String(number=w964) -> (F-format string=w963:string)  [unwired: 3 in]
          }
          frame "MP_THRESHOLD_Y_GYRO_LOW" {
            n440 = Unbundle By Name(w974) -> ("MD_Threshold_References.Y gyro. threshold (L)"=w972:refnum<vi>)
            n441 = property class="DigNum (strict)"(reference=w972, error in=w973) -> (error out=w971:errorcluster, "Value"=w970:dbl)  [unwired: 1 out]
            n442 = Number To Fractional String(number=w970) -> (F-format string=w969:string)  [unwired: 3 in]
          }
          frame "MP_THRESHOLD_Y_GYRO_HIGH" {
            n443 = Unbundle By Name(w980) -> ("MD_Threshold_References.Y gyro. threshold (U)"=w978:refnum<vi>)
            n444 = property class="DigNum (strict)"(reference=w978, error in=w979) -> (error out=w977:errorcluster, "Value"=w976:dbl)  [unwired: 1 out]
            n445 = Number To Fractional String(number=w976) -> (F-format string=w975:string)  [unwired: 3 in]
          }
          frame "MP_THRESHOLD_Z_GYRO_LOW" {
            n446 = Unbundle By Name(w986) -> ("MD_Threshold_References.Z gyro. threshold (L)"=w984:refnum<vi>)
            n447 = property class="DigNum (strict)"(reference=w984, error in=w985) -> (error out=w983:errorcluster, "Value"=w982:dbl)  [unwired: 1 out]
            n448 = Number To Fractional String(number=w982) -> (F-format string=w981:string)  [unwired: 3 in]
          }
          frame "MP_THRESHOLD_Z_GYRO_HIGH" {
            n449 = Unbundle By Name(w992) -> ("MD_Threshold_References.Z gyro. threshold (U)"=w990:refnum<vi>)
            n450 = property class="DigNum (strict)"(reference=w990, error in=w991) -> (error out=w989:errorcluster, "Value"=w988:dbl)  [unwired: 1 out]
            n451 = Number To Fractional String(number=w988) -> (F-format string=w987:string)  [unwired: 3 in]
          }
          frame "MP_THRESHOLD_ROLL_LOW" {
            n452 = Unbundle By Name(w998) -> ("MD_Threshold_References.Roll threshold (L)"=w996:refnum<vi>)
            n453 = property class="DigNum (strict)"(reference=w996, error in=w997) -> (error out=w995:errorcluster, "Value"=w994:dbl)  [unwired: 1 out]
            n454 = Number To Fractional String(number=w994) -> (F-format string=w993:string)  [unwired: 3 in]
          }
          frame "MP_THRESHOLD_ROLL_HIGH" {
            n455 = Unbundle By Name(w1004) -> ("MD_Threshold_References.Roll threshold (U)"=w1002:refnum<vi>)
            n456 = property class="DigNum (strict)"(reference=w1002, error in=w1003) -> (error out=w1001:errorcluster, "Value"=w1000:dbl)  [unwired: 1 out]
            n457 = Number To Fractional String(number=w1000) -> (F-format string=w999:string)  [unwired: 3 in]
          }
          frame "MP_THRESHOLD_PITCH_LOW" {
            n458 = Unbundle By Name(w1010) -> ("MD_Threshold_References.Pitch. threshold (L)"=w1008:refnum<vi>)
            n459 = property class="DigNum (strict)"(reference=w1008, error in=w1009) -> (error out=w1007:errorcluster, "Value"=w1006:dbl)  [unwired: 1 out]
            n460 = Number To Fractional String(number=w1006) -> (F-format string=w1005:string)  [unwired: 3 in]
          }
          frame "MP_THRESHOLD_PITCH_HIGH" {
            n461 = Unbundle By Name(w1016) -> ("MD_Threshold_References.Pitch threshold (U)"=w1014:refnum<vi>)
            n462 = property class="DigNum (strict)"(reference=w1014, error in=w1015) -> (error out=w1013:errorcluster, "Value"=w1012:dbl)  [unwired: 1 out]
            n463 = Number To Fractional String(number=w1012) -> (F-format string=w1011:string)  [unwired: 3 in]
          }
          frame "MP_THRESHOLD_YAW_LOW" {
            n464 = Unbundle By Name(w1022) -> ("MD_Threshold_References.Yaw threshold (L)"=w1020:refnum<vi>)
            n465 = property class="DigNum (strict)"(reference=w1020, error in=w1021) -> (error out=w1019:errorcluster, "Value"=w1018:dbl)  [unwired: 1 out]
            n466 = Number To Fractional String(number=w1018) -> (F-format string=w1017:string)  [unwired: 3 in]
          }
          frame "MP_THRESHOLD_YAW_HIGH" {
            n467 = Unbundle By Name(w1028) -> ("MD_Threshold_References.Yaw threshold (U)"=w1026:refnum<vi>)
            n468 = property class="DigNum (strict)"(reference=w1026, error in=w1027) -> (error out=w1025:errorcluster, "Value"=w1024:dbl)  [unwired: 1 out]
            n469 = Number To Fractional String(number=w1024) -> (F-format string=w1023:string)  [unwired: 3 in]
          }
          frame "MP_DETECTION_TYPE_X_ACCEL" {
            n470 = Unbundle By Name(w1035) -> ("MD_Type_References.X accel threshold type"=w1033:refnum<vi>)
            n471 = property class="Enum (strict)"(reference=w1033, error in=w1034) -> (error out=w1032:errorcluster, "Value"=w1030:T17)  [unwired: 1 out]
            n472 = Index Array(array=string[] ["ABS_LESSER_THAN", "ABS_GREATER_THAN", "LESSER_THAN", "GREATER_THAN", "WINDOWED_MODE_WITHIN_BOUNDS", "WINDOWED_MODE_OUTSIDE_BOUNDS"] ("Array"), index=w1030) -> (element=w1029:string)
          }
          frame "MP_DETECTION_TYPE_Y_ACCEL" {
            n473 = Unbundle By Name(w1042) -> ("MD_Type_References.Y accel threshold type"=w1040:refnum<vi>)
            n474 = property class="Enum (strict)"(reference=w1040, error in=w1041) -> (error out=w1039:errorcluster, "Value"=w1037:T17)  [unwired: 1 out]
            n475 = Index Array(array=string[] ["ABS_LESSER_THAN", "ABS_GREATER_THAN", "LESSER_THAN", "GREATER_THAN", "WINDOWED_MODE_WITHIN_BOUNDS", "WINDOWED_MODE_OUTSIDE_BOUNDS"] ("Array"), index=w1037) -> (element=w1036:string)
          }
          frame "MP_DETECTION_TYPE_Z_ACCEL" {
            n476 = Unbundle By Name(w1049) -> ("MD_Type_References.Z accel threshold type"=w1047:refnum<vi>)
            n477 = property class="Enum (strict)"(reference=w1047, error in=w1048) -> (error out=w1046:errorcluster, "Value"=w1044:T17)  [unwired: 1 out]
            n478 = Index Array(array=string[] ["ABS_LESSER_THAN", "ABS_GREATER_THAN", "LESSER_THAN", "GREATER_THAN", "WINDOWED_MODE_WITHIN_BOUNDS", "WINDOWED_MODE_OUTSIDE_BOUNDS"] ("Array"), index=w1044) -> (element=w1043:string)
          }
          frame "MP_DETECTION_TYPE_X_GYRO" {
            n479 = Unbundle By Name(w1056) -> ("MD_Type_References.X gyro threshold type"=w1054:refnum<vi>)
            n480 = property class="Enum (strict)"(reference=w1054, error in=w1055) -> (error out=w1053:errorcluster, "Value"=w1051:T17)  [unwired: 1 out]
            n481 = Index Array(array=string[] ["ABS_LESSER_THAN", "ABS_GREATER_THAN", "LESSER_THAN", "GREATER_THAN", "WINDOWED_MODE_WITHIN_BOUNDS", "WINDOWED_MODE_OUTSIDE_BOUNDS"] ("Array"), index=w1051) -> (element=w1050:string)
          }
          frame "MP_DETECTION_TYPE_Y_GYRO" {
            n482 = Unbundle By Name(w1063) -> ("MD_Type_References.Y gyro threshold type"=w1061:refnum<vi>)
            n483 = property class="Enum (strict)"(reference=w1061, error in=w1062) -> (error out=w1060:errorcluster, "Value"=w1058:T17)  [unwired: 1 out]
            n484 = Index Array(array=string[] ["ABS_LESSER_THAN", "ABS_GREATER_THAN", "LESSER_THAN", "GREATER_THAN", "WINDOWED_MODE_WITHIN_BOUNDS", "WINDOWED_MODE_OUTSIDE_BOUNDS"] ("Array"), index=w1058) -> (element=w1057:string)
          }
          frame "MP_DETECTION_TYPE_Z_GYRO" {
            n485 = Unbundle By Name(w1070) -> ("MD_Type_References.Z gyro threshold type"=w1068:refnum<vi>)
            n486 = property class="Enum (strict)"(reference=w1068, error in=w1069) -> (error out=w1067:errorcluster, "Value"=w1065:T17)  [unwired: 1 out]
            n487 = Index Array(array=string[] ["ABS_LESSER_THAN", "ABS_GREATER_THAN", "LESSER_THAN", "GREATER_THAN", "WINDOWED_MODE_WITHIN_BOUNDS", "WINDOWED_MODE_OUTSIDE_BOUNDS"] ("Array"), index=w1065) -> (element=w1064:string)
          }
          frame "MP_DETECTION_TYPE_ROLL" {
            n488 = Unbundle By Name(w1077) -> ("MD_Type_References.Roll threshold type"=w1075:refnum<vi>)
            n489 = property class="Enum (strict)"(reference=w1075, error in=w1076) -> (error out=w1074:errorcluster, "Value"=w1072:T17)  [unwired: 1 out]
            n490 = Index Array(array=string[] ["ABS_LESSER_THAN", "ABS_GREATER_THAN", "LESSER_THAN", "GREATER_THAN", "WINDOWED_MODE_WITHIN_BOUNDS", "WINDOWED_MODE_OUTSIDE_BOUNDS"] ("Array"), index=w1072) -> (element=w1071:string)
          }
          frame "MP_DETECTION_TYPE_PITCH" {
            n491 = Unbundle By Name(w1084) -> ("MD_Type_References.Pitch threshold type"=w1082:refnum<vi>)
            n492 = property class="Enum (strict)"(reference=w1082, error in=w1083) -> (error out=w1081:errorcluster, "Value"=w1079:T17)  [unwired: 1 out]
            n493 = Index Array(array=string[] ["ABS_LESSER_THAN", "ABS_GREATER_THAN", "LESSER_THAN", "GREATER_THAN", "WINDOWED_MODE_WITHIN_BOUNDS", "WINDOWED_MODE_OUTSIDE_BOUNDS"] ("Array"), index=w1079) -> (element=w1078:string)
          }
          frame "MP_DETECTION_TYPE_YAW" {
            n494 = Unbundle By Name(w1091) -> ("MD_Type_References.Yaw threshold type"=w1089:refnum<vi>)
            n495 = property class="Enum (strict)"(reference=w1089, error in=w1090) -> (error out=w1088:errorcluster, "Value"=w1086:T17)  [unwired: 1 out]
            n496 = Index Array(array=string[] ["ABS_LESSER_THAN", "ABS_GREATER_THAN", "LESSER_THAN", "GREATER_THAN", "WINDOWED_MODE_WITHIN_BOUNDS", "WINDOWED_MODE_OUTSIDE_BOUNDS"] ("Array"), index=w1086) -> (element=w1085:string)
          }
        }
        n497 = Unbundle By Name(w833) -> ("ADCP"=w835:refnum<vi>)
        n498 = property class="LVClassControl (strict)"(reference=w835) -> (reference out=w834:refnum<vi>, "Value"=w829:refnum<class "ADCP.lvclass">)  [unwired: 1 in, 1 out]
        n499 = call "MPU_Stick_Write_Configuration_Parameter.vi"("ADCP in"=w829, "Parameter Name"=w825, "Parameter Value"=w826, "Write Enable Parameter Name"=w824, "error out"=w830) -> ("ADCP out"=w828:refnum<class "ADCP.lvclass">, "error out"=w827:errorcluster)  [unwired: 8 in, 1 out]
        n500 = property class="LVClassControl (strict)"(reference=w834, "Value"=w828) -> (reference out=w832:refnum<vi>)  [unwired: 1 in, 1 out]
        n501 = Bundle By Name(cluster=w833, "ADCP"=w832) -> (w831:T1)
      }
      frame "Write All" {
        n502 = control-ref of="Configuration Parameter"() -> (w1095:refnum<vi>)
        n503 = property class="Enum (strict)"(reference=w1095, error in=w1097) -> (error out=w1096:errorcluster, "Strings []"=w1093:string[])  [unwired: 1 out]
        n504 = Array Size(array=w1093) -> (size(s)=w1092:i32)
        n505 = for {
          tunnel: w1093 -> [w1123] mode=indexing
          shift-right: [w1124] -> w1099
          shift-left: w1101 -> [w1129]
          shift-right: [w1105] -> w1100
          shift-left: w1096 -> [w1128]
          tunnel: w1098 -> [w1103] mode=indexing
          tunnel: w1094 -> [w1107] mode=indexing
          tunnel: w1092 -> [w1116]
          i -> [w1119]
          n506 = case shown="\"IMU_GYRO_FS\"" w1123 {
            tunnel: w1129 -> [w1134 w1141 w1148 w1155 w1162 w1168 w1174 w1180 w1187 w1194 w1201 w1207 w1213 w1219 w1225 w1231 w1237 w1243 w1249 w1255 w1261 w1267 w1273 w1279 w1285 w1291 w1297 w1303 w1309 w1315 w1321 w1328 w1335 w1342 w1349 w1356 w1363 w1370 w1377 w1384]
            tunnel: [w1134 w1141 w1148 w1155 w1162 w1168 w1174 w1180 w1187 w1194 w1201 w1207 w1213 w1219 w1225 w1231 w1237 w1243 w1249 w1255 w1261 w1267 w1273 w1279 w1285 w1291 w1297 w1303 w1309 w1315 w1321 w1328 w1335 w1342 w1349 w1356 w1363 w1370 w1377 w1384] -> w1122
            tunnel: w1128 -> [w1133 w1140 w1147 w1154 w1161 w1167 w1173 w1179 w1186 w1193 w1200 w1206 w1212 w1218 w1224 w1230 w1236 w1242 w1248 w1254 w1260 w1266 w1272 w1278 w1284 w1290 w1296 w1302 w1308 w1314 w1320 w1327 w1334 w1341 w1348 w1355 w1362 w1369 w1376 w1383]
            tunnel: [w1133 w1138 w1145 w1152 w1159 w1165 w1171 w1177 w1184 w1191 w1198 w1204 w1210 w1216 w1222 w1228 w1234 w1240 w1246 w1252 w1258 w1264 w1270 w1276 w1282 w1288 w1294 w1300 w1306 w1312 w1318 w1325 w1332 w1339 w1346 w1353 w1360 w1367 w1374 w1381] -> w1110
            tunnel: ["" w1135 w1142 w1149 w1157 w1163 w1169 w1175 w1181 w1188 w1195 w1202 w1208 w1214 w1220 w1226 w1232 w1238 w1244 w1250 w1256 w1262 w1268 w1274 w1280 w1286 w1292 w1298 w1304 w1310 w1316 w1322 w1329 w1336 w1343 w1350 w1357 w1364 w1371 w1378] -> w1102
            frame Default {
            }
            frame "IMU_ACCEL_FS" {
              n507 = Unbundle By Name(w1141) -> ("IMU_configuration_references.IMU Accelerometer F.S. value"=w1139:refnum<vi>)
              n508 = property class="Enum (strict)"(reference=w1139, error in=w1140) -> (error out=w1138:errorcluster, "Value"=w1136:T12)  [unwired: 1 out]
              n509 = Index Array(array=string[] ["IMU_ACCEL_FS_2G", "IMU_ACCEL_FS_4G", "IMU_ACCEL_FS_8G", "IMU_ACCEL_FS_16G"], index=w1136) -> (element=w1135:string)
            }
            frame "IMU_ACCEL_BW" {
              n510 = Unbundle By Name(w1148) -> ("IMU_configuration_references.IMU Accelerometer bandwidth"=w1146:refnum<vi>)
              n511 = property class="Enum (strict)"(reference=w1146, error in=w1147) -> (error out=w1145:errorcluster, "Value"=w1144:T13)  [unwired: 1 out]
              n512 = Index Array(array=string[] ["IMU_ACCEL_BW_460Hz", "IMU_ACCEL_BW_184Hz", "IMU_ACCEL_BW_92Hz", "IMU_ACCEL_BW_41Hz", "IMU_ACCEL_BW_20Hz", "IMU_ACCEL_BW_10Hz", "IMU_ACCEL_BW_5Hz"], index=w1144) -> (element=w1142:string)
            }
            frame "IMU_GYRO_FS" {
              n513 = Unbundle By Name(w1155) -> ("IMU_configuration_references.IMU Gyroscope F.S. value"=w1153:refnum<vi>)
              n514 = property class="Enum (strict)"(reference=w1153, error in=w1154) -> (error out=w1152:errorcluster, "Value"=w1151:T14)  [unwired: 1 out]
              n515 = Index Array(array=string[] ["IMU_GYRO_FS_250DPS", "IMU_GYRO_FS_500DPS", "IMU_GYRO_FS_1000DPS", "IMU_GYRO_FS_2000DPS"] ("1D array"), index=w1151) -> (element=w1149:string)
            }
            frame "IMU_GYRO_BW" {
              (unwired) "MPU_STICK:IMU_CONFIG_WRITE_ENABLE:IMU_CONFIG_GYRO_BW_WE"
              n516 = Unbundle By Name(w1162) -> ("IMU_configuration_references.IMU Gyroscope bandwidth"=w1160:refnum<vi>)
              n517 = property class="Enum (strict)"(reference=w1160, error in=w1161) -> (error out=w1159:errorcluster, "Value"=w1158:T15)  [unwired: 1 out]
              n518 = Index Array(array=string[] ["IMU_GYRO_BW_NONE", "IMU_GYRO_BW_184Hz", "IMU_GYRO_BW_92Hz", "IMU_GYRO_BW_41Hz", "IMU_GYRO_BW_20Hz", "IMU_GYRO_BW_10Hz", "IMU_GYRO_BW_5Hz"] ("1D array"), index=w1158) -> (element=w1157:string)
            }
            frame "IMU_CALIB_INTERVAL" {
              n519 = Unbundle By Name(w1168) -> ("IMU_configuration_references.Calibration interval (ms)"=w1166:refnum<vi>)
              n520 = property class="DigNum (strict)"(reference=w1166, error in=w1167) -> (error out=w1165:errorcluster, "Value"=w1164:u16)  [unwired: 1 out]
              n521 = Number To Decimal String(number=w1164) -> (decimal integer string=w1163:string)  [unwired: 1 in]
            }
            frame "IMU_CALIB_POINT_COUNT" {
              n522 = Unbundle By Name(w1174) -> ("IMU_configuration_references.Calibration point count"=w1172:refnum<vi>)
              n523 = property class="DigNum (strict)"(reference=w1172, error in=w1173) -> (error out=w1171:errorcluster, "Value"=w1170:u16)  [unwired: 1 out]
              n524 = Number To Decimal String(number=w1170) -> (decimal integer string=w1169:string)  [unwired: 1 in]
            }
            frame "IMU_SAMPLING_FREQ" {
              n525 = Unbundle By Name(w1180) -> ("IMU_configuration_references.Sampling frequency (Hz)"=w1178:refnum<vi>)
              n526 = property class="DigNum (strict)"(reference=w1178, error in=w1179) -> (error out=w1177:errorcluster, "Value"=w1176:u16)  [unwired: 1 out]
              n527 = Number To Decimal String(number=w1176) -> (decimal integer string=w1175:string)  [unwired: 1 in]
            }
            frame "LED1_CONFIG" {
              n528 = Unbundle By Name(w1187) -> ("LED_Configuration_References.LED1 Configuration"=w1185:refnum<vi>)
              n529 = property class="Enum (strict)"(reference=w1185, error in=w1186) -> (error out=w1184:errorcluster, "Value"=w1182:T16)  [unwired: 1 out]
              n530 = Index Array(array=string[] ["USER_CONTROLLED_DIG_OUTPUT", "X_ACCEL_PWM", "Y_ACCEL_PWM", "Z_ACCEL_PWM", "X_ACCEL_MD_OUTPUT", "Y_ACCEL_MD_OUTPUT", "Z_ACCEL_MD_OUTPUT", "X_GYRO_PWM", "Y_ACCEL_PWM", "Z_ACCEL_PWM", "X_GYRO_MD_OUTPUT", "Y_GYRO_MD_OUTPUT", "Z_GYRO_MD_OUTPUT", "ROLL_PWM", "PITCH_PWM", "YAW_PWM", "ROLL_MD_OUTPUT", "PITCH_MD_OUTPUT", "YAW_MD_OUTPUT", "USER_CONTROLLED_PWM_OUTPUT"] ("Array"), index=w1182) -> (element=w1181:string)
            }
            frame "LED2_CONFIG" {
              n531 = Unbundle By Name(w1194) -> ("LED_Configuration_References.LED2 Configuration"=w1192:refnum<vi>)
              n532 = property class="Enum (strict)"(reference=w1192, error in=w1193) -> (error out=w1191:errorcluster, "Value"=w1189:T16)  [unwired: 1 out]
              n533 = Index Array(array=string[] ["USER_CONTROLLED_DIG_OUTPUT", "X_ACCEL_PWM", "Y_ACCEL_PWM", "Z_ACCEL_PWM", "X_ACCEL_MD_OUTPUT", "Y_ACCEL_MD_OUTPUT", "Z_ACCEL_MD_OUTPUT", "X_GYRO_PWM", "Y_ACCEL_PWM", "Z_ACCEL_PWM", "X_GYRO_MD_OUTPUT", "Y_GYRO_MD_OUTPUT", "Z_GYRO_MD_OUTPUT", "ROLL_PWM", "PITCH_PWM", "YAW_PWM", "ROLL_MD_OUTPUT", "PITCH_MD_OUTPUT", "YAW_MD_OUTPUT", "USER_CONTROLLED_PWM_OUTPUT"] ("Array"), index=w1189) -> (element=w1188:string)
            }
            frame "LED3_CONFIG" {
              n534 = Unbundle By Name(w1201) -> ("LED_Configuration_References.LED3 Configuration"=w1199:refnum<vi>)
              n535 = property class="Enum (strict)"(reference=w1199, error in=w1200) -> (error out=w1198:errorcluster, "Value"=w1196:T16)  [unwired: 1 out]
              n536 = Index Array(array=string[] ["USER_CONTROLLED_DIG_OUTPUT", "X_ACCEL_PWM", "Y_ACCEL_PWM", "Z_ACCEL_PWM", "X_ACCEL_MD_OUTPUT", "Y_ACCEL_MD_OUTPUT", "Z_ACCEL_MD_OUTPUT", "X_GYRO_PWM", "Y_ACCEL_PWM", "Z_ACCEL_PWM", "X_GYRO_MD_OUTPUT", "Y_GYRO_MD_OUTPUT", "Z_GYRO_MD_OUTPUT", "ROLL_PWM", "PITCH_PWM", "YAW_PWM", "ROLL_MD_OUTPUT", "PITCH_MD_OUTPUT", "YAW_MD_OUTPUT", "USER_CONTROLLED_PWM_OUTPUT"] ("Array"), index=w1196) -> (element=w1195:string)
            }
            frame "MP_ROLL_FILTER_CONSTANT" {
              n537 = Unbundle By Name(w1207) -> ("MP_Comp_Filter_Constants_References.Roll filter constant"=w1205:refnum<vi>)
              n538 = property class="DigNum (strict)"(reference=w1205, error in=w1206) -> (error out=w1204:errorcluster, "Value"=w1203:dbl)  [unwired: 1 out]
              n539 = Number To Fractional String(number=w1203) -> (F-format string=w1202:string)  [unwired: 3 in]
            }
            frame "MP_PITCH_FILTER_CONSTANT" {
              n540 = Unbundle By Name(w1213) -> ("MP_Comp_Filter_Constants_References.Pitch filter constant"=w1211:refnum<vi>)
              n541 = property class="DigNum (strict)"(reference=w1211, error in=w1212) -> (error out=w1210:errorcluster, "Value"=w1209:dbl)  [unwired: 1 out]
              n542 = Number To Fractional String(number=w1209) -> (F-format string=w1208:string)  [unwired: 3 in]
            }
            frame "MP_THRESHOLD_X_ACCEL_LOW" {
              n543 = Unbundle By Name(w1219) -> ("MD_Threshold_References.X accel. threshold (L)"=w1217:refnum<vi>)
              n544 = property class="DigNum (strict)"(reference=w1217, error in=w1218) -> (error out=w1216:errorcluster, "Value"=w1215:dbl)  [unwired: 1 out]
              n545 = Number To Fractional String(number=w1215) -> (F-format string=w1214:string)  [unwired: 3 in]
            }
            frame "MP_THRESHOLD_X_ACCEL_HIGH" {
              n546 = Unbundle By Name(w1225) -> ("MD_Threshold_References.X accel. threshold (U)"=w1223:refnum<vi>)
              n547 = property class="DigNum (strict)"(reference=w1223, error in=w1224) -> (error out=w1222:errorcluster, "Value"=w1221:dbl)  [unwired: 1 out]
              n548 = Number To Fractional String(number=w1221) -> (F-format string=w1220:string)  [unwired: 3 in]
            }
            frame "MP_THRESHOLD_Y_ACCEL_LOW" {
              n549 = Unbundle By Name(w1231) -> ("MD_Threshold_References.Y accel. threshold (L)"=w1229:refnum<vi>)
              n550 = property class="DigNum (strict)"(reference=w1229, error in=w1230) -> (error out=w1228:errorcluster, "Value"=w1227:dbl)  [unwired: 1 out]
              n551 = Number To Fractional String(number=w1227) -> (F-format string=w1226:string)  [unwired: 3 in]
            }
            frame "MP_THRESHOLD_Y_ACCEL_HIGH" {
              n552 = Unbundle By Name(w1237) -> ("MD_Threshold_References.Y accel. threshold (U)"=w1235:refnum<vi>)
              n553 = property class="DigNum (strict)"(reference=w1235, error in=w1236) -> (error out=w1234:errorcluster, "Value"=w1233:dbl)  [unwired: 1 out]
              n554 = Number To Fractional String(number=w1233) -> (F-format string=w1232:string)  [unwired: 3 in]
            }
            frame "MP_THRESHOLD_Z_ACCEL_LOW" {
              n555 = Unbundle By Name(w1243) -> ("MD_Threshold_References.Z accel. threshold (L)"=w1241:refnum<vi>)
              n556 = property class="DigNum (strict)"(reference=w1241, error in=w1242) -> (error out=w1240:errorcluster, "Value"=w1239:dbl)  [unwired: 1 out]
              n557 = Number To Fractional String(number=w1239) -> (F-format string=w1238:string)  [unwired: 3 in]
            }
            frame "MP_THRESHOLD_Z_ACCEL_HIGH" {
              n558 = Unbundle By Name(w1249) -> ("MD_Threshold_References.Z accel. threshold (U)"=w1247:refnum<vi>)
              n559 = property class="DigNum (strict)"(reference=w1247, error in=w1248) -> (error out=w1246:errorcluster, "Value"=w1245:dbl)  [unwired: 1 out]
              n560 = Number To Fractional String(number=w1245) -> (F-format string=w1244:string)  [unwired: 3 in]
            }
            frame "MP_THRESHOLD_X_GYRO_LOW" {
              n561 = Unbundle By Name(w1255) -> ("MD_Threshold_References.X gyro. threshold (L)"=w1253:refnum<vi>)
              n562 = property class="DigNum (strict)"(reference=w1253, error in=w1254) -> (error out=w1252:errorcluster, "Value"=w1251:dbl)  [unwired: 1 out]
              n563 = Number To Fractional String(number=w1251) -> (F-format string=w1250:string)  [unwired: 3 in]
            }
            frame "MP_THRESHOLD_X_GYRO_HIGH" {
              n564 = Unbundle By Name(w1261) -> ("MD_Threshold_References.X gyro. threshold (U)"=w1259:refnum<vi>)
              n565 = property class="DigNum (strict)"(reference=w1259, error in=w1260) -> (error out=w1258:errorcluster, "Value"=w1257:dbl)  [unwired: 1 out]
              n566 = Number To Fractional String(number=w1257) -> (F-format string=w1256:string)  [unwired: 3 in]
            }
            frame "MP_THRESHOLD_Y_GYRO_LOW" {
              n567 = Unbundle By Name(w1267) -> ("MD_Threshold_References.Y gyro. threshold (L)"=w1265:refnum<vi>)
              n568 = property class="DigNum (strict)"(reference=w1265, error in=w1266) -> (error out=w1264:errorcluster, "Value"=w1263:dbl)  [unwired: 1 out]
              n569 = Number To Fractional String(number=w1263) -> (F-format string=w1262:string)  [unwired: 3 in]
            }
            frame "MP_THRESHOLD_Y_GYRO_HIGH" {
              n570 = Unbundle By Name(w1273) -> ("MD_Threshold_References.Y gyro. threshold (U)"=w1271:refnum<vi>)
              n571 = property class="DigNum (strict)"(reference=w1271, error in=w1272) -> (error out=w1270:errorcluster, "Value"=w1269:dbl)  [unwired: 1 out]
              n572 = Number To Fractional String(number=w1269) -> (F-format string=w1268:string)  [unwired: 3 in]
            }
            frame "MP_THRESHOLD_Z_GYRO_LOW" {
              n573 = Unbundle By Name(w1279) -> ("MD_Threshold_References.Z gyro. threshold (L)"=w1277:refnum<vi>)
              n574 = property class="DigNum (strict)"(reference=w1277, error in=w1278) -> (error out=w1276:errorcluster, "Value"=w1275:dbl)  [unwired: 1 out]
              n575 = Number To Fractional String(number=w1275) -> (F-format string=w1274:string)  [unwired: 3 in]
            }
            frame "MP_THRESHOLD_Z_GYRO_HIGH" {
              n576 = Unbundle By Name(w1285) -> ("MD_Threshold_References.Z gyro. threshold (U)"=w1283:refnum<vi>)
              n577 = property class="DigNum (strict)"(reference=w1283, error in=w1284) -> (error out=w1282:errorcluster, "Value"=w1281:dbl)  [unwired: 1 out]
              n578 = Number To Fractional String(number=w1281) -> (F-format string=w1280:string)  [unwired: 3 in]
            }
            frame "MP_THRESHOLD_ROLL_LOW" {
              n579 = Unbundle By Name(w1291) -> ("MD_Threshold_References.Roll threshold (L)"=w1289:refnum<vi>)
              n580 = property class="DigNum (strict)"(reference=w1289, error in=w1290) -> (error out=w1288:errorcluster, "Value"=w1287:dbl)  [unwired: 1 out]
              n581 = Number To Fractional String(number=w1287) -> (F-format string=w1286:string)  [unwired: 3 in]
            }
            frame "MP_THRESHOLD_ROLL_HIGH" {
              n582 = Unbundle By Name(w1297) -> ("MD_Threshold_References.Roll threshold (U)"=w1295:refnum<vi>)
              n583 = property class="DigNum (strict)"(reference=w1295, error in=w1296) -> (error out=w1294:errorcluster, "Value"=w1293:dbl)  [unwired: 1 out]
              n584 = Number To Fractional String(number=w1293) -> (F-format string=w1292:string)  [unwired: 3 in]
            }
            frame "MP_THRESHOLD_PITCH_LOW" {
              n585 = Unbundle By Name(w1303) -> ("MD_Threshold_References.Pitch. threshold (L)"=w1301:refnum<vi>)
              n586 = property class="DigNum (strict)"(reference=w1301, error in=w1302) -> (error out=w1300:errorcluster, "Value"=w1299:dbl)  [unwired: 1 out]
              n587 = Number To Fractional String(number=w1299) -> (F-format string=w1298:string)  [unwired: 3 in]
            }
            frame "MP_THRESHOLD_PITCH_HIGH" {
              n588 = Unbundle By Name(w1309) -> ("MD_Threshold_References.Pitch threshold (U)"=w1307:refnum<vi>)
              n589 = property class="DigNum (strict)"(reference=w1307, error in=w1308) -> (error out=w1306:errorcluster, "Value"=w1305:dbl)  [unwired: 1 out]
              n590 = Number To Fractional String(number=w1305) -> (F-format string=w1304:string)  [unwired: 3 in]
            }
            frame "MP_THRESHOLD_YAW_LOW" {
              n591 = Unbundle By Name(w1315) -> ("MD_Threshold_References.Yaw threshold (L)"=w1313:refnum<vi>)
              n592 = property class="DigNum (strict)"(reference=w1313, error in=w1314) -> (error out=w1312:errorcluster, "Value"=w1311:dbl)  [unwired: 1 out]
              n593 = Number To Fractional String(number=w1311) -> (F-format string=w1310:string)  [unwired: 3 in]
            }
            frame "MP_THRESHOLD_YAW_HIGH" {
              n594 = Unbundle By Name(w1321) -> ("MD_Threshold_References.Yaw threshold (U)"=w1319:refnum<vi>)
              n595 = property class="DigNum (strict)"(reference=w1319, error in=w1320) -> (error out=w1318:errorcluster, "Value"=w1317:dbl)  [unwired: 1 out]
              n596 = Number To Fractional String(number=w1317) -> (F-format string=w1316:string)  [unwired: 3 in]
            }
            frame "MP_DETECTION_TYPE_X_ACCEL" {
              n597 = Unbundle By Name(w1328) -> ("MD_Type_References.X accel threshold type"=w1326:refnum<vi>)
              n598 = property class="Enum (strict)"(reference=w1326, error in=w1327) -> (error out=w1325:errorcluster, "Value"=w1323:T17)  [unwired: 1 out]
              n599 = Index Array(array=string[] ["ABS_LESSER_THAN", "ABS_GREATER_THAN", "LESSER_THAN", "GREATER_THAN", "WINDOWED_MODE_WITHIN_BOUNDS", "WINDOWED_MODE_OUTSIDE_BOUNDS"] ("Array"), index=w1323) -> (element=w1322:string)
            }
            frame "MP_DETECTION_TYPE_Y_ACCEL" {
              n600 = Unbundle By Name(w1335) -> ("MD_Type_References.Y accel threshold type"=w1333:refnum<vi>)
              n601 = property class="Enum (strict)"(reference=w1333, error in=w1334) -> (error out=w1332:errorcluster, "Value"=w1330:T17)  [unwired: 1 out]
              n602 = Index Array(array=string[] ["ABS_LESSER_THAN", "ABS_GREATER_THAN", "LESSER_THAN", "GREATER_THAN", "WINDOWED_MODE_WITHIN_BOUNDS", "WINDOWED_MODE_OUTSIDE_BOUNDS"] ("Array"), index=w1330) -> (element=w1329:string)
            }
            frame "MP_DETECTION_TYPE_Z_ACCEL" {
              n603 = Unbundle By Name(w1342) -> ("MD_Type_References.Z accel threshold type"=w1340:refnum<vi>)
              n604 = property class="Enum (strict)"(reference=w1340, error in=w1341) -> (error out=w1339:errorcluster, "Value"=w1337:T17)  [unwired: 1 out]
              n605 = Index Array(array=string[] ["ABS_LESSER_THAN", "ABS_GREATER_THAN", "LESSER_THAN", "GREATER_THAN", "WINDOWED_MODE_WITHIN_BOUNDS", "WINDOWED_MODE_OUTSIDE_BOUNDS"] ("Array"), index=w1337) -> (element=w1336:string)
            }
            frame "MP_DETECTION_TYPE_X_GYRO" {
              n606 = Unbundle By Name(w1349) -> ("MD_Type_References.X gyro threshold type"=w1347:refnum<vi>)
              n607 = property class="Enum (strict)"(reference=w1347, error in=w1348) -> (error out=w1346:errorcluster, "Value"=w1344:T17)  [unwired: 1 out]
              n608 = Index Array(array=string[] ["ABS_LESSER_THAN", "ABS_GREATER_THAN", "LESSER_THAN", "GREATER_THAN", "WINDOWED_MODE_WITHIN_BOUNDS", "WINDOWED_MODE_OUTSIDE_BOUNDS"] ("Array"), index=w1344) -> (element=w1343:string)
            }
            frame "MP_DETECTION_TYPE_Y_GYRO" {
              n609 = Unbundle By Name(w1356) -> ("MD_Type_References.Y gyro threshold type"=w1354:refnum<vi>)
              n610 = property class="Enum (strict)"(reference=w1354, error in=w1355) -> (error out=w1353:errorcluster, "Value"=w1351:T17)  [unwired: 1 out]
              n611 = Index Array(array=string[] ["ABS_LESSER_THAN", "ABS_GREATER_THAN", "LESSER_THAN", "GREATER_THAN", "WINDOWED_MODE_WITHIN_BOUNDS", "WINDOWED_MODE_OUTSIDE_BOUNDS"] ("Array"), index=w1351) -> (element=w1350:string)
            }
            frame "MP_DETECTION_TYPE_Z_GYRO" {
              n612 = Unbundle By Name(w1363) -> ("MD_Type_References.Z gyro threshold type"=w1361:refnum<vi>)
              n613 = property class="Enum (strict)"(reference=w1361, error in=w1362) -> (error out=w1360:errorcluster, "Value"=w1358:T17)  [unwired: 1 out]
              n614 = Index Array(array=string[] ["ABS_LESSER_THAN", "ABS_GREATER_THAN", "LESSER_THAN", "GREATER_THAN", "WINDOWED_MODE_WITHIN_BOUNDS", "WINDOWED_MODE_OUTSIDE_BOUNDS"] ("Array"), index=w1358) -> (element=w1357:string)
            }
            frame "MP_DETECTION_TYPE_ROLL" {
              n615 = Unbundle By Name(w1370) -> ("MD_Type_References.Roll threshold type"=w1368:refnum<vi>)
              n616 = property class="Enum (strict)"(reference=w1368, error in=w1369) -> (error out=w1367:errorcluster, "Value"=w1365:T17)  [unwired: 1 out]
              n617 = Index Array(array=string[] ["ABS_LESSER_THAN", "ABS_GREATER_THAN", "LESSER_THAN", "GREATER_THAN", "WINDOWED_MODE_WITHIN_BOUNDS", "WINDOWED_MODE_OUTSIDE_BOUNDS"] ("Array"), index=w1365) -> (element=w1364:string)
            }
            frame "MP_DETECTION_TYPE_PITCH" {
              n618 = Unbundle By Name(w1377) -> ("MD_Type_References.Pitch threshold type"=w1375:refnum<vi>)
              n619 = property class="Enum (strict)"(reference=w1375, error in=w1376) -> (error out=w1374:errorcluster, "Value"=w1372:T17)  [unwired: 1 out]
              n620 = Index Array(array=string[] ["ABS_LESSER_THAN", "ABS_GREATER_THAN", "LESSER_THAN", "GREATER_THAN", "WINDOWED_MODE_WITHIN_BOUNDS", "WINDOWED_MODE_OUTSIDE_BOUNDS"] ("Array"), index=w1372) -> (element=w1371:string)
            }
            frame "MP_DETECTION_TYPE_YAW" {
              n621 = Unbundle By Name(w1384) -> ("MD_Type_References.Yaw threshold type"=w1382:refnum<vi>)
              n622 = property class="Enum (strict)"(reference=w1382, error in=w1383) -> (error out=w1381:errorcluster, "Value"=w1379:T17)  [unwired: 1 out]
              n623 = Index Array(array=string[] ["ABS_LESSER_THAN", "ABS_GREATER_THAN", "LESSER_THAN", "GREATER_THAN", "WINDOWED_MODE_WITHIN_BOUNDS", "WINDOWED_MODE_OUTSIDE_BOUNDS"] ("Array"), index=w1379) -> (element=w1378:string)
            }
          }
          n624 = To Double Precision Float(number=w1116) -> (double precision float=w1115:dbl)
          n625 = Increment(x=w1119) -> (x+1=w1118:i32)
          n626 = To Double Precision Float(number=w1118) -> (double precision float=w1117:dbl)
          n627 = Divide(x=w1117, y=w1115) -> (x/y=w1114:dbl)
          n628 = Multiply(x=100.0, y=w1114) -> (x*y=w1112:dbl)
          n629 = To Unsigned Byte Integer(number=w1112) -> (unsigned 8bit integer=w1111:u8)
          n630 = Unbundle By Name(w1122) -> ("Primary_references.Progress Bar"=w1121:refnum<vi>)
          n631 = property class="Slide (strict)"(reference=w1121, "Value"=w1111, "Caption.Text"="Writing all configurations") -> ()  [unwired: 1 in, 2 out]
          n632 = Unbundle By Name(w1122) -> ("ADCP"=w1127:refnum<vi>)
          n633 = property class="LVClassControl (strict)"(reference=w1127) -> (reference out=w1126:refnum<vi>, "Value"=w1109:refnum<class "ADCP.lvclass">)  [unwired: 1 in, 1 out]
          n634 = call "MPU_Stick_Write_Configuration_Parameter.vi"("ADCP in"=w1109, "Parameter Name"=w1103, "Parameter Value"=w1102, "Write Enable Parameter Name"=w1107, "error out"=w1110) -> ("ADCP out"=w1108:refnum<class "ADCP.lvclass">, "Result"=w1104:bool, "error out"=w1106:errorcluster)  [unwired: 8 in]
          n635 = case shown="False" w1104 {
            tunnel: w1106 -> [w1130 w1131]
            tunnel: [w1130 w1131] -> w1105
            frame False {
            }
            frame True {
            }
          }
          n636 = property class="LVClassControl (strict)"(reference=w1126, "Value"=w1108) -> (reference out=w1125:refnum<vi>)  [unwired: 1 in, 1 out]
          n637 = Bundle By Name(cluster=w1122, "ADCP"=w1125) -> (w1124:T1)
        }
      }
    }
  }
  "error out" <- w2
  "MPU_Stick_Globals Out" <- w1
